vi "simple-LevyLab Analysis Framework (Template).vi"() -> ()   [LabVIEW 2019]
doc: "simple-LevyLab Analysis Framework (s-LLAF).\n\nDrag onto an empty block diagram to make your own."
uses:
  <vilib>/PRIrvin/XY Utilities/Typedefs/Interpolation Configuration--cluster.ctl
  <userlib>/LevyLab/LV-Data/LV-Data.ITX/Typedefs/Retrieve Data Type.ctl
  <vilib>/PRIrvin/Graph Utilities/graph_utilities.lvclass
  <userlib>/LevyLab/LV-Data/LV-Data/Typedefs/Dictionary--cluster.ctl
  <vilib>/PRIrvin/Graph Utilities/graph_utilities.lvclass/graph_utilities.ctl
  c6ffbd9c-2039-4b06-9ae2-0340eb0d4766.vi
  <vilib>/Analysis/baseanly.llb/Mean (DBL).vi
  4205ac38-1c06-43f0-93e0-ac3005b12872.vi
  <vilib>/Analysis/baseanly.llb/A x B.vi
  <vilib>/Analysis/baseanly.llb/A x Vector.vi
  <vilib>/PRIrvin/XY Utilities/subVIs/Square (single).vi
  <vilib>/PRIrvin/XY Utilities/subVIs/Sort (single).vi
  <vilib>/PRIrvin/XY Utilities/subVIs/Decimate (single).vi
  <vilib>/PRIrvin/XY Utilities/subVIs/Swap X and Y (single).vi
  <vilib>/PRIrvin/XY Utilities/subVIs/Reverse (single).vi
  <vilib>/PRIrvin/XY Utilities/subVIs/Subset (single).vi
  <vilib>/PRIrvin/XY Utilities/subVIs/Derivative (single).vi
  <vilib>/PRIrvin/XY Utilities/subVIs/Difference Quotient (single).vi
  <vilib>/PRIrvin/XY Utilities/subVIs/Interpolate (single).vi
  <vilib>/PRIrvin/XY Utilities/subVIs/FFT (single).vi
  <vilib>/PRIrvin/XY Utilities/subVIs/PS (single).vi
  <vilib>/PRIrvin/XY Utilities/subVIs/Moving Average (single).vi
  <vilib>/PRIrvin/XY Utilities/subVIs/Savitsky Golay Filter (single).vi
  <vilib>/PRIrvin/XY Utilities/subVIs/Zero Phase Lowpass Filter (single).vi
  <vilib>/PRIrvin/XY Utilities/subVIs/Symmetrize (single).vi
  <vilib>/Analysis/2dsp.llb/Decimate (single shot).vi
  <vilib>/Analysis/2dsp.llb/Decimate (single shot, DBL).vi
  <vilib>/Analysis/2dsp.llb/Derivative x(t).vi
  <vilib>/PRIrvin/XY Utilities/Private/X Array Index to Range.vi
  <vilib>/PRIrvin/XY Utilities/Private/X Units.vi
  <vilib>/PRIrvin/XY Utilities/Private/DQ subVI.vi
  <vilib>/PRIrvin/XY Utilities/subVIs/Divide float (single).vi
  <vilib>/PRIrvin/XY Utilities/subVIs/Add XY (single).vi
  <vilib>/PRIrvin/XY Utilities/subVIs/XY to Waveform (single).vi
  <vilib>/PRIrvin/XY Utilities/Private/Get X Array dx.vi
  <vilib>/Analysis/3filter.llb/Savitzky-Golay Filter.vi
  <vilib>/Analysis/3filter.llb/Savitzky-Golay Filter (DBL).vi
  <vilib>/PRIrvin/XY Utilities/Private/X Array Range to Index.vi
  <vilib>/PRIrvin/XY Utilities/subVIs/Get X and Y (single).vi
  <vilib>/PRIrvin/XY Utilities/subVIs/Resample (single).vi
  <vilib>/PRIrvin/Graph Utilities/XY Graph/Set XY Graph Value (array).vi
  <vilib>/PRIrvin/Graph Utilities/XY Graph/Get XY Graph Value.vi
  <vilib>/PRIrvin/Graph Utilities/Intensity Graph/Set Intensity Graph X Scale Array.vi
  <vilib>/PRIrvin/Graph Utilities/XY Graph/Get XY Graph X Label.vi
  <vilib>/PRIrvin/Graph Utilities/Intensity Graph/Set Intensity Graph X Label.vi
  <vilib>/PRIrvin/Graph Utilities/XY Graph/Get XY Graph Y Label.vi
  <vilib>/PRIrvin/Graph Utilities/Intensity Graph/Set Intensity Graph Z Label.vi
  <vilib>/PRIrvin/Graph Utilities/Intensity Graph/Set Intensity Graph Y Scale Array.vi
  <vilib>/PRIrvin/Graph Utilities/Intensity Graph/Set Intensity Graph Y Label.vi
  <vilib>/PRIrvin/Graph Utilities/Intensity Graph/Get Intensity Graph Cursor (Control).vi
  <vilib>/PRIrvin/Graph Utilities/Intensity Graph/Set Intensity Graph Cursor.vi
  <vilib>/PRIrvin/Graph Utilities/Intensity Graph/Get Intensity Graph X Scale.vi
  <vilib>/PRIrvin/Graph Utilities/Intensity Graph/Get Intensity Graph Value.vi
  <vilib>/PRIrvin/Graph Utilities/Intensity Graph/Get Intensity Graph Y Scale.vi
  <vilib>/PRIrvin/Graph Utilities/subVIs/Step Average.vi
  <vilib>/PRIrvin/Graph Utilities/subVIs/Normalized Gaussian.vi
  <vilib>/PRIrvin/Graph Utilities/Intensity Graph/Get Intensity Graph Y Label.vi
  <vilib>/PRIrvin/Graph Utilities/XY Graph/Set XY Graph X Label.vi
  <vilib>/PRIrvin/Graph Utilities/Intensity Graph/Get Intensity Graph Z Label.vi
  <vilib>/PRIrvin/Graph Utilities/XY Graph/Set XY Graph Y Label.vi
  <vilib>/PRIrvin/Graph Utilities/Intensity Graph/Get Intensity Graph X Label.vi
  <userlib>/_OpenG.lib/file/file.llb/Build Path - File Names Array__ogtk.vi
  <userlib>/_OpenG.lib/array/array.llb/Sort Array__ogtk.vi
  <userlib>/_OpenG.lib/array/array.llb/Sort 1D Array (DBL)__ogtk.vi
  <userlib>/_OpenG.lib/array/array.llb/Reorder Array2__ogtk.vi
  <userlib>/_OpenG.lib/array/array.llb/Reorder 1D Array2 (DBL)__ogtk.vi
  <userlib>/_MGI/1D Array/MGI Interpolate 1D Array Extended.vi
  <vilib>/Analysis/1siggen.llb/Ramp Pattern.vi
  <vilib>/Analysis/1siggen.llb/Ramp Pattern by Delta.vi
  <vilib>/gmath/interp.llb/Interpolate 1D.vi
  <vilib>/measure/maresamp.llb/Resample Waveforms (single shot).vi
  <vilib>/measure/maresamp.llb/Resample Pair of Arrays (single shot).vi
  <vilib>/measure/maspectr.llb/FFT Spectrum (Mag-Phase).vi
  <vilib>/measure/maspectr.llb/FFT Spectrum (Mag-Phase) for 1 Chan.vi
  <vilib>/measure/maspectr.llb/FFT Power Spectrum and PSD.vi
  <vilib>/measure/maspectr.llb/FFT Power Spectrum and PSD for 1 Chan.vi
  <vilib>/measure/maresamp.llb/Resample N Pairs of Arrays (single shot).vi
  <vilib>/ptbypt/Probability & Statistics.llb/Mean PtByPt.vi
  <vilib>/Analysis/3filter.llb/FIR Windowed Coefficients.vi
  <vilib>/Analysis/3filter.llb/Zero Phase Filter.vi
  <vilib>/Analysis/3filter.llb/Zero Phase Filter (DBL).vi
  <vilib>/PRIrvin/XY Utilities/xy_utilities.lvlib
  <userlib>/LevyLab/LV-Data/LV-Data/LV-Data.lvclass
  <userlib>/LevyLab/LV-Data/LV-Data.ITX/LV-Data.ITX.lvclass
  <vilib>/Analysis/NI_AALBase.lvlib
  <userlib>/LevyLab/LV-Data/LV-Data/API/XY-Data to Dictionary (single).vi
  <vilib>/PRIrvin/XY Utilities/subVIs/Subtract float (single).vi
  <vilib>/PRIrvin/XY Utilities/subVIs/Add float (single).vi
  <vilib>/PRIrvin/XY Utilities/subVIs/Waveform to XY (single).vi
  <vilib>/PRIrvin/XY Utilities/subVIs/Multiply float (single).vi
  <vilib>/PRIrvin/XY Utilities/subVIs/Restrict X Range (single).vi
  <vilib>/PRIrvin/XY Utilities/subVIs/Interpolate Y (single).vi
  <vilib>/PRIrvin/XY Utilities/subVIs/Log (single).vi
  <vilib>/PRIrvin/XY Utilities/subVIs/Linear Fit (multiple).vi
  <vilib>/PRIrvin/XY Utilities/subVIs/Append (multiple).vi
  <vilib>/PRIrvin/XY Utilities/subVIs/Shift Zero (single).vi
  <vilib>/PRIrvin/XY Utilities/subVIs/Peak Detector (single).vi
  <vilib>/PRIrvin/XY Utilities/subVIs/Remove Outliers (single).vi
  a4d1e059-db4b-46df-9b26-41dcdcc29953.vi
  8d1aee34-a274-4619-8160-c9a8fc862039.vi
  eec88c9d-a91b-41fb-93d9-32a34acbf560.vi
  a819f7a0-c833-4e57-b12c-b555cdea62a2.vi
  2a0ce4de-3a5e-4348-8ae1-e372722f1305.vi
  8311829f-ef70-43ef-acfd-10b322ed8a94.vi
  <vilib>/PRIrvin/XY Utilities/subVIs/Add float (multiple).vi
  <vilib>/PRIrvin/XY Utilities/subVIs/Subtract float (multiple).vi
  <vilib>/PRIrvin/XY Utilities/subVIs/Multiply float (multiple).vi
  <vilib>/PRIrvin/XY Utilities/subVIs/Square (multiple).vi
  <vilib>/PRIrvin/XY Utilities/subVIs/Divide float (multiple).vi
  <vilib>/PRIrvin/XY Utilities/subVIs/Sort (multiple).vi
  <vilib>/PRIrvin/XY Utilities/subVIs/Decimate (multiple).vi
  <vilib>/PRIrvin/XY Utilities/subVIs/Swap X and Y (multiple).vi
  <vilib>/PRIrvin/XY Utilities/subVIs/Reverse (multiple).vi
  <vilib>/PRIrvin/XY Utilities/subVIs/Subset (multiple).vi
  <vilib>/PRIrvin/XY Utilities/subVIs/Derivative (multiple).vi
  <vilib>/PRIrvin/XY Utilities/subVIs/Difference Quotient (multiple).vi
  <vilib>/PRIrvin/XY Utilities/subVIs/Interpolate (multiple).vi
  <vilib>/PRIrvin/XY Utilities/subVIs/FFT (multiple).vi
  <vilib>/PRIrvin/XY Utilities/subVIs/PS (multiple).vi
  <vilib>/PRIrvin/XY Utilities/subVIs/Resample (multiple).vi
  <vilib>/PRIrvin/XY Utilities/subVIs/Moving Average (multiple).vi
  <vilib>/PRIrvin/XY Utilities/subVIs/Savitsky Golay Filter (multiple).vi
  <vilib>/PRIrvin/XY Utilities/subVIs/Zero Phase Lowpass Filter (multiple).vi
  <vilib>/PRIrvin/XY Utilities/subVIs/Symmetrize (multiple).vi
panel:
  out "time (ms)":dbl
  in  "Tab Control":enum32{"Load Data", "Help"}(tab)
  in  "regex after":string
  in  "param in notes":bool
  in  "list recursive":bool
  in  "Path":path
  out "Notes":string
  in  "Data Type":T1=enum."DAT"
  in  "SAVE":bool
  in  "PROCESS":bool
  in  "CLEAR":bool
  in  "LOAD":bool
  in  "Z":u16(ring) items=["Delay", "Temperature", "Time", "Ch1_x", "Ch1_y", "Ch1_PS_x", "Ch1_PS_y", "Ch2_x", "Ch2_y", "Ch2_PS_x", "Ch2_PS_y", "Ch3_x", "Ch3_y", "Ch3_PS_x", "Ch3_PS_y", "Ch4_x", "Ch4_y", "Ch4_PS_x", "Ch4_PS_y", "Ch5_x", "Ch5_y", "Ch5_PS_x", "Ch5_PS_y", "Ch6_x", "Ch6_y", "Ch6_PS_x", "Ch6_PS_y", "Ch7_x", "Ch7_y", "Ch7_PS_x", "Ch7_PS_y", "Ch8_x", "Ch8_y", "Ch8_PS_x", "Ch8_PS_y"]
  in  "Y":u16(ring) items=["Delay", "Temperature", "Time", "Ch1_x", "Ch1_y", "Ch1_PS_x", "Ch1_PS_y", "Ch2_x", "Ch2_y", "Ch2_PS_x", "Ch2_PS_y", "Ch3_x", "Ch3_y", "Ch3_PS_x", "Ch3_PS_y", "Ch4_x", "Ch4_y", "Ch4_PS_x", "Ch4_PS_y", "Ch5_x", "Ch5_y", "Ch5_PS_x", "Ch5_PS_y", "Ch6_x", "Ch6_y", "Ch6_PS_x", "Ch6_PS_y", "Ch7_x", "Ch7_y", "Ch7_PS_x", "Ch7_PS_y", "Ch8_x", "Ch8_y", "Ch8_PS_x", "Ch8_PS_y"]
  in  "A":u16(ring) items=["Delay", "Temperature", "Time", "Ch1_x", "Ch1_y", "Ch1_PS_x", "Ch1_PS_y", "Ch2_x", "Ch2_y", "Ch2_PS_x", "Ch2_PS_y", "Ch3_x", "Ch3_y", "Ch3_PS_x", "Ch3_PS_y", "Ch4_x", "Ch4_y", "Ch4_PS_x", "Ch4_PS_y", "Ch5_x", "Ch5_y", "Ch5_PS_x", "Ch5_PS_y", "Ch6_x", "Ch6_y", "Ch6_PS_x", "Ch6_PS_y", "Ch7_x", "Ch7_y", "Ch7_PS_x", "Ch7_PS_y", "Ch8_x", "Ch8_y", "Ch8_PS_x", "Ch8_PS_y"]
  in  "C":u16(ring) items=["Delay", "Temperature", "Time", "Ch1_x", "Ch1_y", "Ch1_PS_x", "Ch1_PS_y", "Ch2_x", "Ch2_y", "Ch2_PS_x", "Ch2_PS_y", "Ch3_x", "Ch3_y", "Ch3_PS_x", "Ch3_PS_y", "Ch4_x", "Ch4_y", "Ch4_PS_x", "Ch4_PS_y", "Ch5_x", "Ch5_y", "Ch5_PS_x", "Ch5_PS_y", "Ch6_x", "Ch6_y", "Ch6_PS_x", "Ch6_PS_y", "Ch7_x", "Ch7_y", "Ch7_PS_x", "Ch7_PS_y", "Ch8_x", "Ch8_y", "Ch8_PS_x", "Ch8_PS_y"]
  in  "B":u16(ring) items=["Delay", "Temperature", "Time", "Ch1_x", "Ch1_y", "Ch1_PS_x", "Ch1_PS_y", "Ch2_x", "Ch2_y", "Ch2_PS_x", "Ch2_PS_y", "Ch3_x", "Ch3_y", "Ch3_PS_x", "Ch3_PS_y", "Ch4_x", "Ch4_y", "Ch4_PS_x", "Ch4_PS_y", "Ch5_x", "Ch5_y", "Ch5_PS_x", "Ch5_PS_y", "Ch6_x", "Ch6_y", "Ch6_PS_x", "Ch6_PS_y", "Ch7_x", "Ch7_y", "Ch7_PS_x", "Ch7_PS_y", "Ch8_x", "Ch8_y", "Ch8_PS_x", "Ch8_PS_y"]
  in  "X":u16(ring) items=["Delay", "Temperature", "Time", "Ch1_x", "Ch1_y", "Ch1_PS_x", "Ch1_PS_y", "Ch2_x", "Ch2_y", "Ch2_PS_x", "Ch2_PS_y", "Ch3_x", "Ch3_y", "Ch3_PS_x", "Ch3_PS_y", "Ch4_x", "Ch4_y", "Ch4_PS_x", "Ch4_PS_y", "Ch5_x", "Ch5_y", "Ch5_PS_x", "Ch5_PS_y", "Ch6_x", "Ch6_y", "Ch6_PS_x", "Ch6_PS_y", "Ch7_x", "Ch7_y", "Ch7_PS_x", "Ch7_PS_y", "Ch8_x", "Ch8_y", "Ch8_PS_x", "Ch8_PS_y"]
  in  "regex before":string
  in  "Action Tab Control":enum32{"Page 1", "Page 2"}(tab)
  out "Processed States":string="XY: Load\nGraph: Initialize Graphs\nUI: Display Data"
  in  "Available States":i32(listbox)=-1 caption="States to Process"
  in  "Process Queue":string
  out "Current State":string
  in  "Type":enum16{"y/x vs x", "x/y vs y"}(ring)
  in  "Window":dbl=2.0
  in  "Units":enum16{"Points", "Data"}(ring)
  in  "Configure":T2={"X Low"=0.05, "X High"=0.5, "X Step"=0.01, "Fake Point"=0.05} {"Fake Point" format="%#_6p"; "X Step" format="%#_6p"; "X High" format="%#_6p"; "X Low" format="%#_6p"}
  in  "y":dbl format="%#_6p"
  in  "x":dbl format="%#_6p"
  in  "Type":enum16{"dy/dx vs x", "dx/dy vs y"}(ring)
  in  "Subset Slider":cluster{dbl, dbl}(slide)={0.75, 0.25} caption="Horizontal Slider" scale=0.0..1.0
  in  "Method":enum16{"Slider (%)", "X[] min and max"}(ring)
  in  "SG side points":dbl
  in  "Moving Window":dbl=5000.0 format="%#_13g"
  in  "Zero Phase cutoff":dbl
  in  "decimating factor":i32=1
  in  "averaging":bool
  in  "Graphs Tab Control":enum32{"Data", "Intensity/Linecuts"}(tab)
  out "XY Graph: Antisymmetric":cluster{"X-array":dbl[], dbl[]}[](graph)
  out "XY Graph: Processed":cluster{"Intensity Data":dbl[], "Array":dbl[]}[](graph)
  out "XY Graph: Unprocessed":cluster{"Intensity Data":dbl[], "Array":dbl[]}[](graph)
  out "XY Graph: Symmetric":cluster{"X-array":dbl[], dbl[]}[](graph)
  out "Data Intensity":dbl[][](graph)
  out "Diff Intensity":dbl[][](graph)
  out "Diff Vertical":cluster{"Array":dbl[], "A x Vector":dbl[]}[](graph)
  out "Diff Horizontal":cluster{"Array":dbl[], "A x Vector":dbl[]}[](graph)
  in  "width (vertical)":dbl=0.2 caption="width"
  in  "width (horizontal)":dbl=0.2 caption="width"
  in  "width (vertical) 2":dbl=0.2 caption="width"
  in  "width (horizontal) 2":dbl=0.2 caption="width"
  out "Data Vertical":cluster{"Array":dbl[], "A x Vector":dbl[]}[](graph)
  out "Data Horizontal":cluster{"Intensity Data":dbl[], "Array":dbl[]}[](graph)
  in  "Color Map":T3(ring)=enum."Viridis"
  in  "Color Map 2":T3(ring)=enum."Viridis"
  # "Load Data"
  # "Actions"
  # "Load Data:\n- \"Path\" can be a file or a folder; \"TDMS Groups\" will read this many groups from a single file\n- A,B,C refer to the 1st, 2nd, 3rd datasets to read from the file. They are combined in the state \"Data: Select Channels\" to calculate, for example Rxx or Rxy\n- X, Y, Z are independent vaiables (eg, X = Vsg, Y = Magnet)\nState Scripting:\n- \"Process Queue\" is a list of states that will execute when you press the \"PROCESS\" button. (File: Load and Graph: Update Graph are added automatically to the beginning and end of the queue.)\nTo add states you can either:\n- Type directly into the Process Queue box.\nor:\n- Select a state in the \"Available States\" box that you want to add to the queue. ctl-v in the \"Process Queue\" control to add to the queue."
  # "State Scripting"
  # "Process Arguments"
  # "Arithmetic"
  # "Interpolate"
  # "Subset"
  # "Filters"
  # "Derivative"
  # "Difference Quotient"
  # "XY Graphs"
  # "Symmeterized Graphs"
  # "Data processing (1)"
  # "Data Processing (2)"
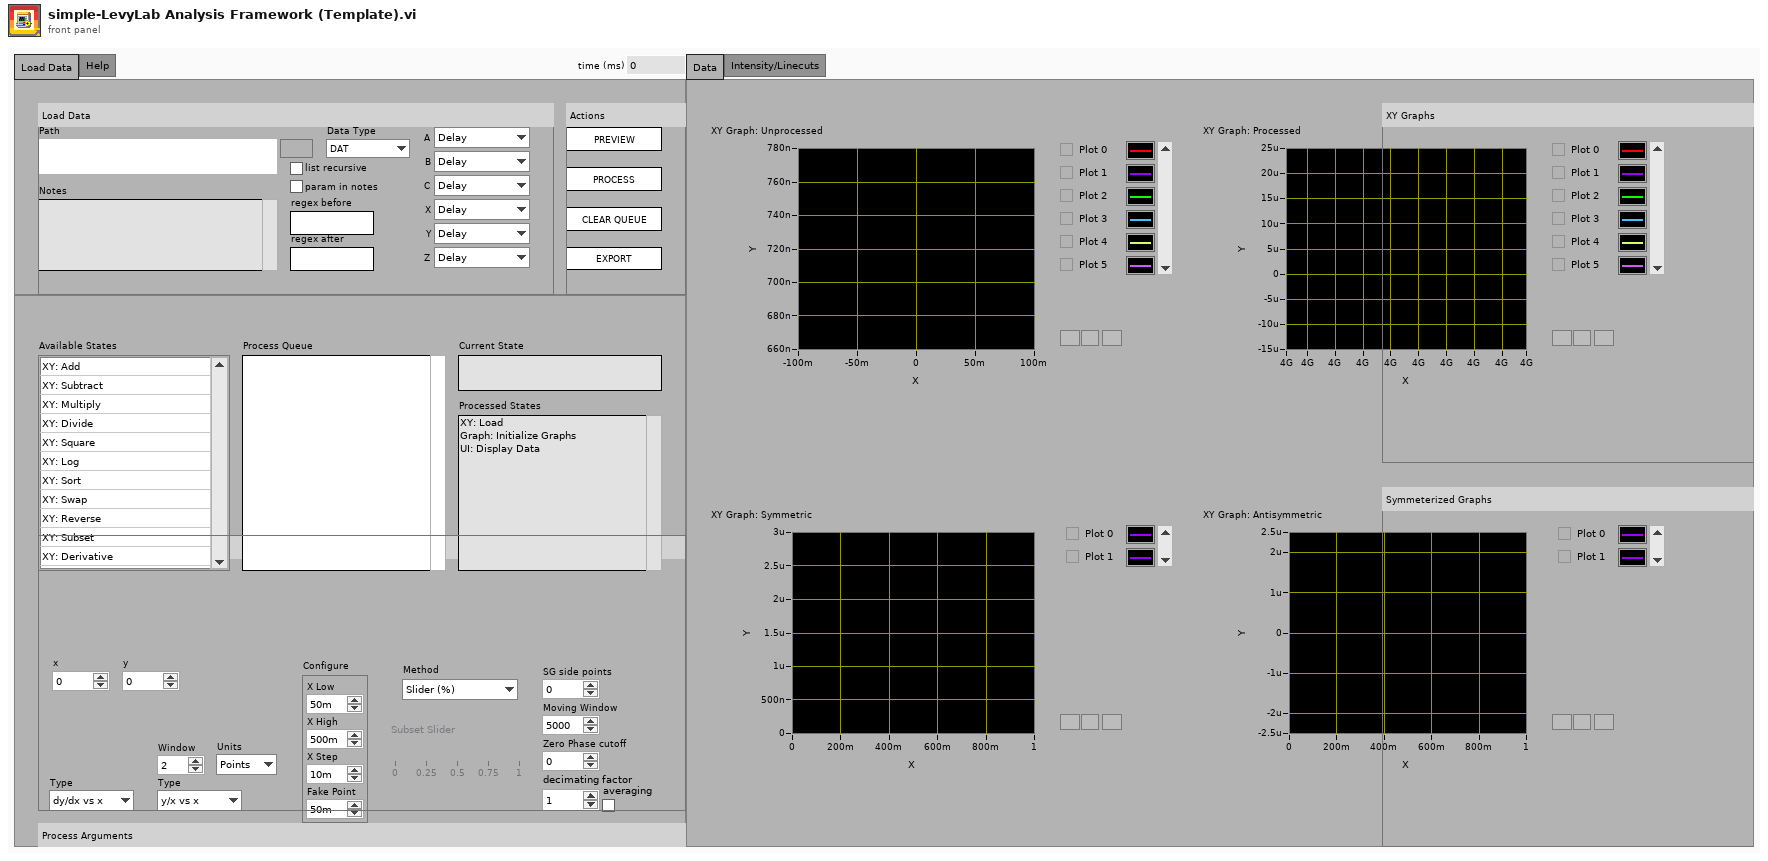
[diagram p1: front panel]
types:
  T1 = typedef "LV-Data.ITX.lvclass/Retrieve Data Type.ctl" = enum16{"ITX", "ITX w/ 2D", "DAT", "TDMS"}
  T2 = typedef "xy_utilities.lvlib/Interpolation Configuration--cluster.ctl" = cluster{"X Low":dbl, "X High":dbl, "X Step":dbl, "Fake Point":dbl}
  T3 = enum16{"Inferno", "Kindlmann", "Plasma", "Viridis", "LevyLab2010", "ColorCET...", "Custom..."}
  T4 = enum32{"Invalid", "Standard", "Closed", "Hidden", "Minimized", "Maximized"}
  T5 = enum32{"invalid app kind", "Development System", "Run Time System", "Student Edition", "Embedded LabVIEW", "Evaluation", "Custom"}
  T6 = typedef "LV-Data.lvclass/Dictionary--cluster.ctl" = cluster{"key":string, "value":variant}
  T7 = cluster{"Core":cluster{"Current VI Reference":refnum<vi>, "Close Panel on Exit?":bool}, "Path":path, "Paths":path[], "Graph":cluster{"Data: Unprocessed":refnum<class "graph_utilities.lvclass">, "Data: Processed":refnum<class "graph_utilities.lvclass">, "Data: Intensity/Vertical":refnum<class "graph_utilities.lvclass">, "Data: Intensity/Horizontal":refnum<class "graph_utilities.lvclass">, "Differential: Intensity/Vertical":refnum<class "graph_utilities.lvclass">, "Differential: Intensity/Horizontal":refnum<class "graph_utilities.lvclass">}, "Rings":cluster{"X":refnum<vi>, "Y":refnum<vi>, "Z":refnum<vi>, "A":refnum<vi>, "B":refnum<vi>, "C":refnum<vi>}, "Dictionaries":cluster{"Data (Dictionary)":T6[]}[], "Keys":cluster{"X":string, "Y":string, "Z":string, "A":string, "B":string, "C":string}, "XY Data (unprocessed)":cluster{"X-array":dbl[], "Y-array":dbl[]}[], "XY Data (processed 1)":cluster{"X-array":dbl[], "Y-array":dbl[]}[], "XY Data (processed 2)":cluster{"X-array":dbl[], "Y-array":dbl[]}[], "Parameter":dbl[]}
  T8 = cluster{"Shift":bool, "Ctrl":bool, "Alt":bool, "Cmd":bool, "Opt":bool}
  T9 = cluster{"X":string, "Y":string, "Z":string, "A":string, "B":string, "C":string}
  T10 = cluster{"X":refnum<vi>, "Y":refnum<vi>, "Z":refnum<vi>, "A":refnum<vi>, "B":refnum<vi>, "C":refnum<vi>}
  T11 = cluster{"Data: Unprocessed":refnum<class "graph_utilities.lvclass">, "Data: Processed":refnum<class "graph_utilities.lvclass">, "Data: Intensity/Vertical":refnum<class "graph_utilities.lvclass">, "Data: Intensity/Horizontal":refnum<class "graph_utilities.lvclass">, "Differential: Intensity/Vertical":refnum<class "graph_utilities.lvclass">, "Differential: Intensity/Horizontal":refnum<class "graph_utilities.lvclass">}
  T12 = cluster{"Current VI Reference":refnum<vi>, "Close Panel on Exit?":bool}
  T13 = typedef "LV-Data.lvclass/Map Variant--map.ctl" = map{string, variant}
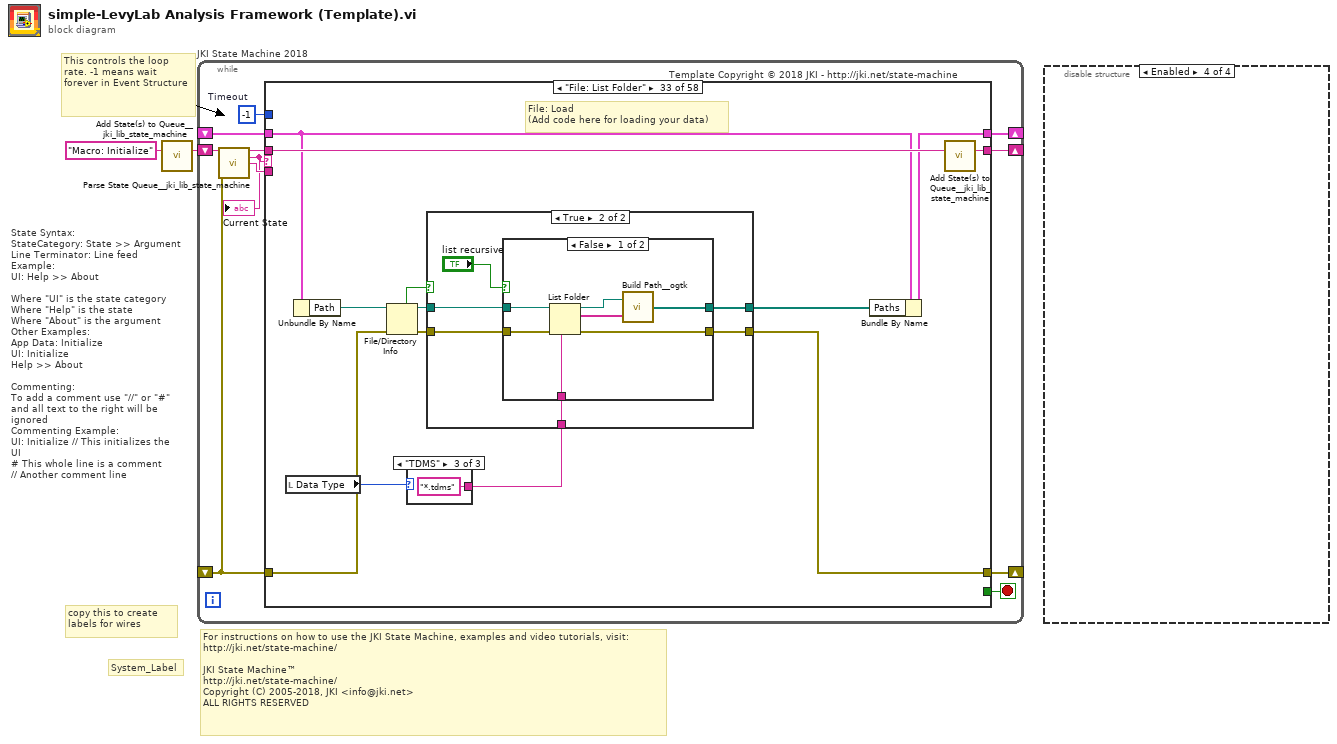
[diagram p0: block diagram]
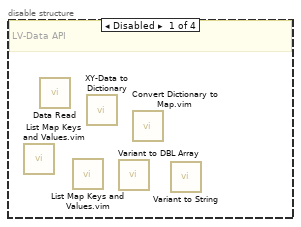
[diagram p2: hidden frame]
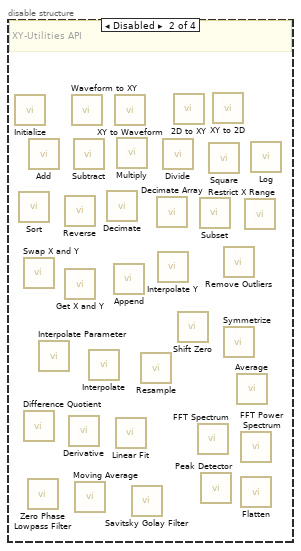
[diagram p3: hidden frame]
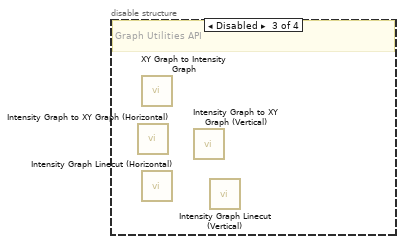
[diagram p4: hidden frame]
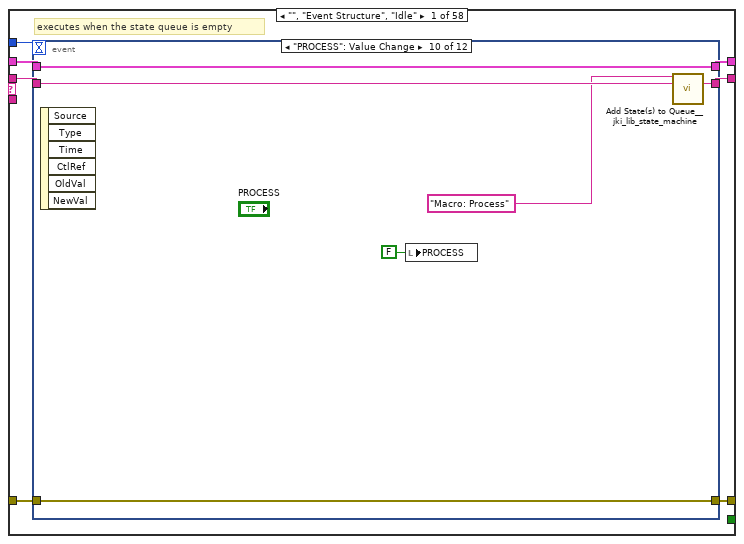
[diagram p5: hidden frame]
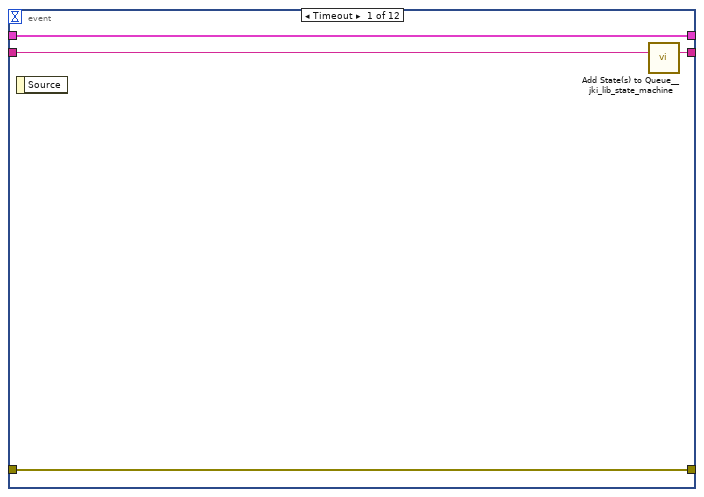
[diagram p6: hidden frame]
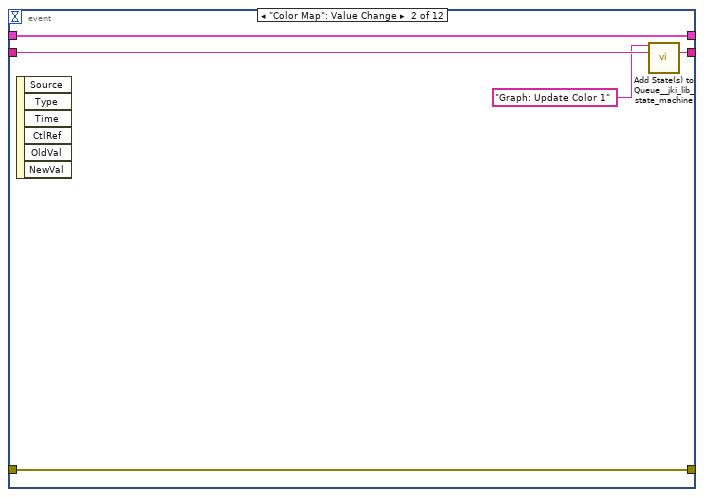
[diagram p7: hidden frame]
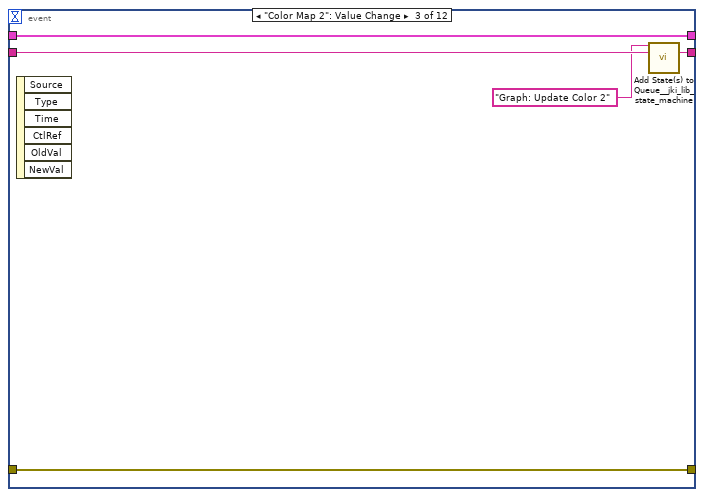
[diagram p8: hidden frame]
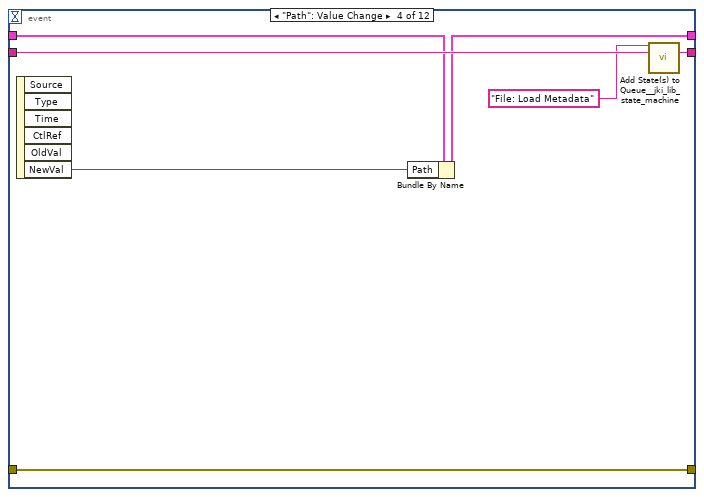
[diagram p9: hidden frame]
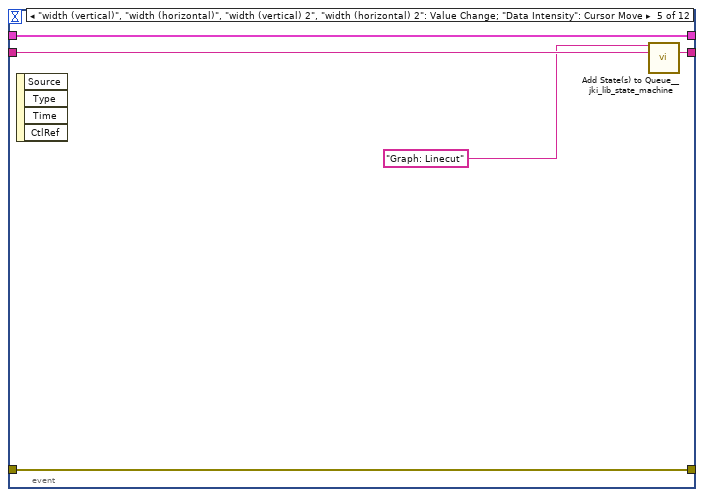
[diagram p10: hidden frame]
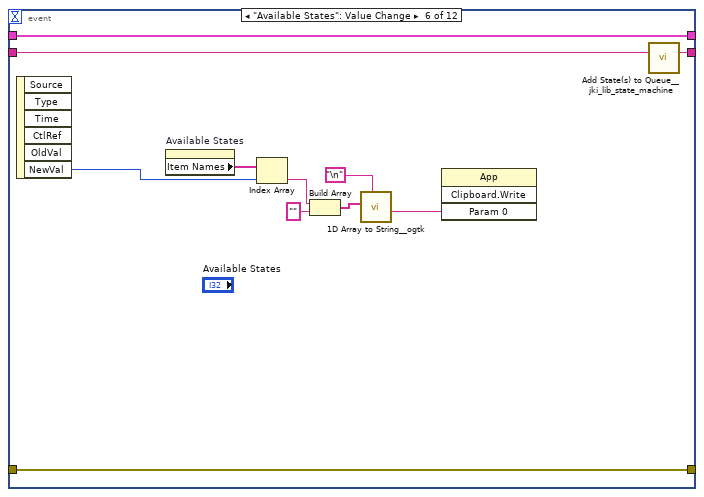
[diagram p11: hidden frame]
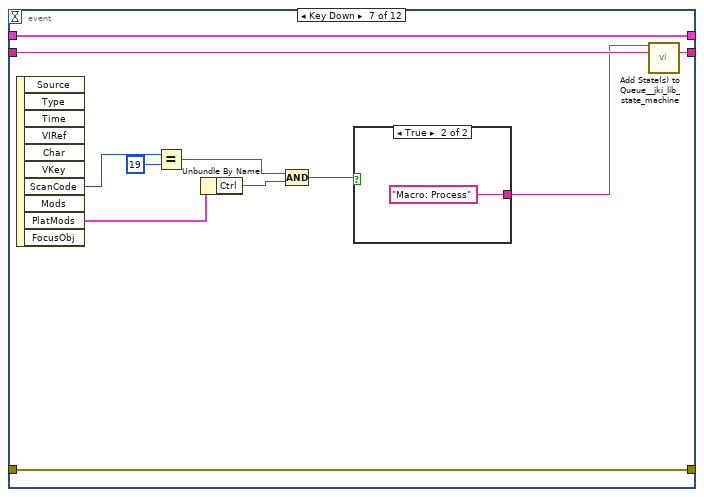
[diagram p12: hidden frame]
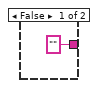
[diagram p13: hidden frame]
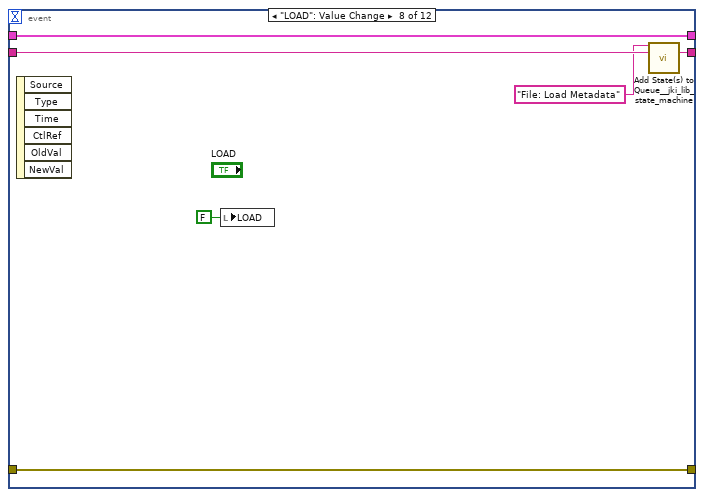
[diagram p14: hidden frame]
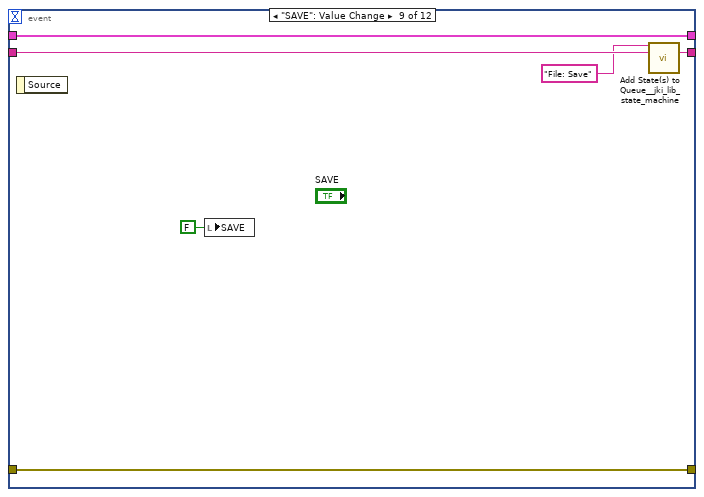
[diagram p15: hidden frame]
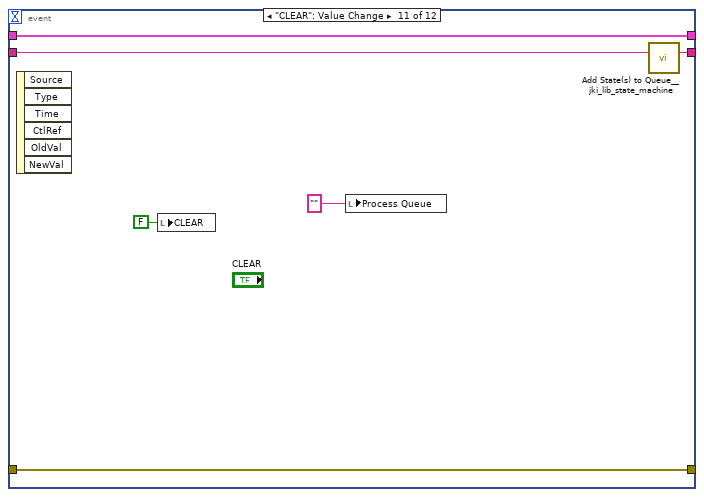
[diagram p16: hidden frame]
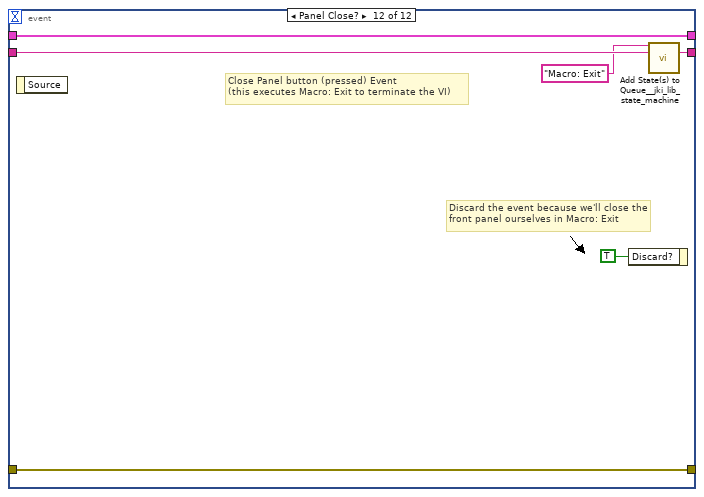
[diagram p17: hidden frame]
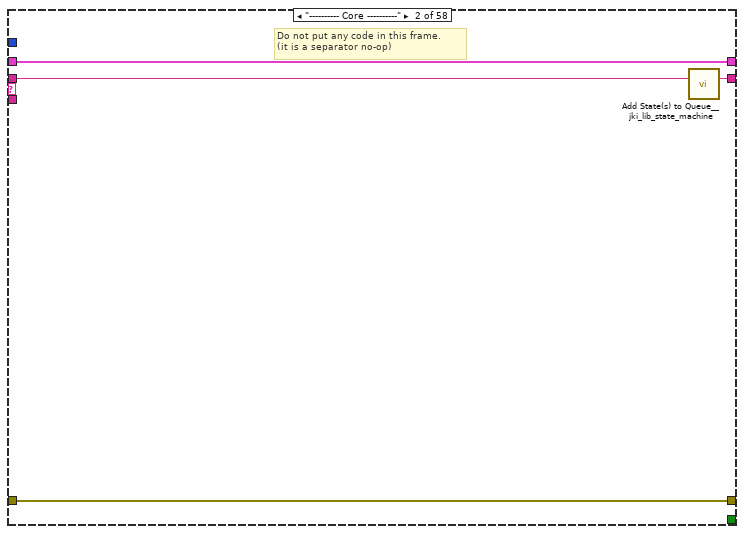
[diagram p18: hidden frame]
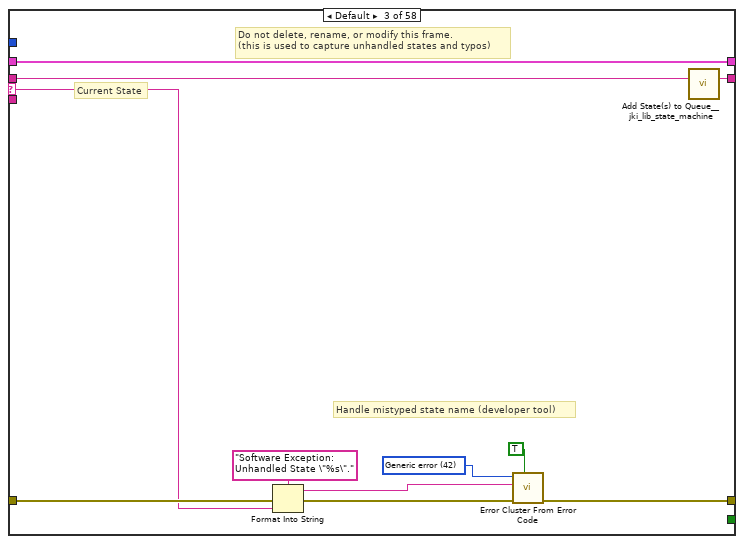
[diagram p19: hidden frame]
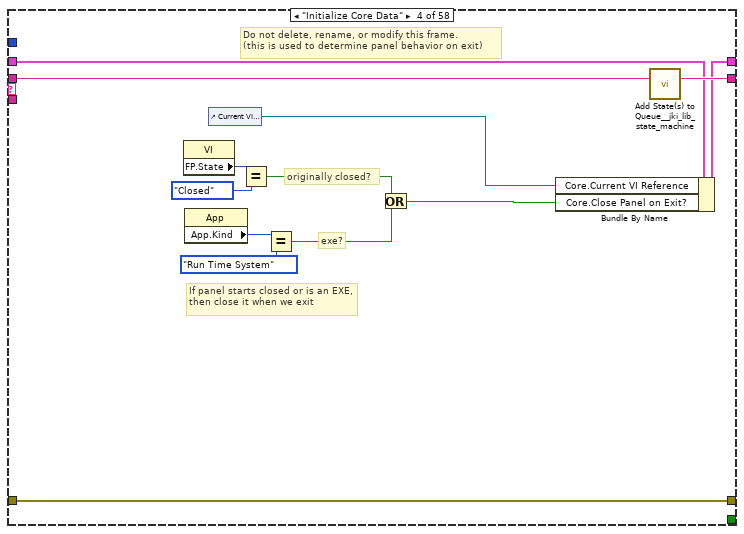
[diagram p20: hidden frame]
diagram:
  # "For instructions on how to use the JKI State Machine, examples and video tutorials, visit:\nhttp://jki.net/state-machine/\n\nJKI State Machine™\nhttp://jki.net/state-machine/\nCopyright (C) 2005-2018, JKI <info@jki.net>\nALL RIGHTS RESERVED"
  # "State Syntax:\nStateCategory: State >> Argument\nLine Terminator: Line feed\nExample:\nUI: Help >> About\n\nWhere \"UI\" is the state category\nWhere \"Help\" is the state\nWhere \"About\" is the argument\nOther Examples:\nApp Data: Initialize\nUI: Initialize\nHelp >> About\n\nCommenting:\nTo add a comment use \"//\" or \"#\" and all text to the right will be ignored\nCommenting Example:\nUI: Initialize // This initializes the UI\n# This whole line is a comment\n// Another comment line"
  # "copy this to create labels for wires"
  # "This controls the loop rate. -1 means wait forever in Event Structure"
  # "System_Label"
  n1 = call <vilib>:"Add State(s) to Queue__jki_lib_state_machine.vi"("State(s) in (\"\")"="Macro: Initialize") -> ("States Out"=w2:string)  [unwired: 14 in]
  n2 = while "JKI State Machine 2018" {
    shift-right: [w7] -> _
    shift-left: _ -> [w6]
    shift-right: [w10] -> _
    shift-left: _ -> [w4]
    shift-right: [w9] -> _
    shift-left: w2 -> [w11]
    stop <- w8 stop-if-true
    w5 = -1  # Timeout
    # "Template Copyright © 2018 JKI - http://jki.net/state-machine"
    n3 = call <vilib>:"Parse State Queue__jki_lib_state_machine.vi"("State Queue"=w11, "Error In (no error)"=w4) -> ("Remaining States"=w13:string, "Current State"=w3:string, "Arguments"=w12:string)  [unwired: 11 in]
    "Current State" <- w3
    n4 = case shown="\"File: List Folder\"" w3 {
      selector: w3 -> [_ _ w105 _ _ _ _ _ _ _ _ _ _ _ _ _ _ _ _ _ _ _ _ _ _ _ _ _ _ _ _ _ _ _ _ _ _ _ _ _ _ _ _ _ _ _ _ _ _ _ _ _ _ _ _ _ _ _]
      tunnel: w13 -> [w20 w104 w109 w128 w134 w139 w143 w158 w173 w191 w226 w230 w242 w248 w259 w328 w333 w343 w353 w357 w361 w378 w402 w413 w423 w450 w485 w501 w509 w517 w521 w538 w579 w614 w653 w661 w671 w681 w691 w699 w706 w720 w728 w738 w746 w754 w765 w778 w789 w798 w806 w814 w822 w830 w839 w848 w857 w867]
      tunnel: w12 -> [_ _ _ _ _ _ _ _ _ _ _ _ _ w243 w253 _ _ _ _ _ _ _ _ _ _ _ _ _ _ _ _ _ _ _ _ _ _ _ _ _ _ _ _ _ _ _ w755 _ _ _ _ _ _ _ _ _ _ _]
      tunnel: w6 -> [w18 w101 w107 w121 w131 w137 w140 _ w166 w187 w221 w227 w240 w246 w255 w325 w330 w340 w350 w354 w358 w376 w400 w409 w420 w448 w482 w499 w507 w515 w518 w536 w576 w611 w650 w658 w668 w678 w688 w696 w704 w717 w725 w735 w743 w751 w762 w775 w786 w795 w803 w811 w819 w827 w836 w845 w854 w864]
      tunnel: [w17 w102 w111 w125 errorcluster {"status"=FALSE, "code"=0, "source"=""} ("error out") w136 w141 w155 w160 w186 w222 w228 w233 w244 w256 w326 w331 w341 w351 w355 w359 w374 w385 w411 w418 w440 w483 w490 w503 w512 w519 w530 w568 w605 w648 w654 w664 w674 w684 w692 w702 w713 w721 w731 w739 w747 w758 w772 w783 w791 w799 w808 w815 w823 w832 w841 w850 w860] -> w10
      tunnel: w4 -> [w16 w102 w110 w125 w130 w136 w141 w155 w168 w183 w223 w228 w234 w245 w257 w326 w331 w341 w351 w355 w359 w365 w379 w411 w419 w443 w483 w492 w502 w511 w519 w526 w574 w606 w647 w655 w665 w675 w685 w693 w702 w714 w722 w732 w740 w748 w759 w773 w784 w792 w800 w809 w816 w824 w833 w842 w851 w861]
      tunnel: [w19 w103 w108 w127 w133 w138 w142 w157 w172 w190 w225 w229 w241 w247 w258 w327 w332 w342 w352 w356 w360 w377 w401 w412 w422 w449 w484 w500 w508 w516 w520 w537 w578 w613 w652 w660 w670 w680 w690 w698 w705 w719 w727 w737 w745 w753 w764 w777 w788 w797 w805 w813 w821 w829 w838 w847 w856 w866] -> w9
      tunnel: [_ _ _ _ _ TRUE _ _ _ _ _ _ _ _ _ _ _ _ _ _ _ _ _ _ _ _ _ _ _ _ _ _ _ _ _ _ _ _ _ _ _ _ _ _ _ _ _ _ _ _ _ _ _ _ _ _ _ _] -> w8
      tunnel: [w15 w101 w107 w126 w131 w137 w140 w156 w167 w188 w221 w227 w240 w246 w255 w325 w330 w340 w350 w354 w358 w375 w399 w410 w420 w448 w482 w499 w507 w515 w518 w536 w577 w612 w650 w657 w667 w677 w687 w695 w703 w716 w724 w734 w742 w750 w761 w774 w785 w794 w802 w810 w818 w826 w835 w844 w853 w863] -> w7
      tunnel: w5 -> [w14 _ _ _ _ _ _ _ _ _ _ _ _ _ _ _ _ _ _ _ _ _ _ _ _ _ _ _ _ _ _ _ _ _ _ _ _ _ _ _ _ _ _ _ _ _ _ _ _ _ _ _ _ _ _ _ _ _]
      frame "", "Event Structure", "Idle" {
        # "executes when the state queue is empty"
        n5 = event shown="[9] \"PROCESS\": Value Change" {
          selector: _ -> [_ _ _ _ _ _ _ _ _ _ _ _]
          dyn-events: _ -> [_ _ _ _ _ _ _ _ _ _ _ _]
          timeout: w14 -> [_ _ _ _ _ _ _ _ _ _ _ _]
          tunnel: w20 -> [w24 w29 w34 w41 w46 w57 w68 w76 w82 w88 w94 w100]
          tunnel: [w23 w28 w33 w40 w45 w56 w67 w75 w81 w87 w93 w99] -> w19
          tunnel: w18 -> [w21 w26 w31 w37 w43 w54 w65 w73 w79 w85 w91 w97]
          tunnel: [w22 w27 w32 w39 w44 w55 w66 w74 w80 w86 w92 w98] -> w17
          tunnel: w16 -> [w22 w27 w32 w39 w44 w55 w66 w74 w80 w86 w92 w98]
          tunnel: [w21 w26 w31 w38 w43 w54 w65 w73 w79 w85 w91 w97] -> w15
          event Timeout {
            n6 = event-data() -> ()  [unwired: 1 in, 1 out]
            n7 = call <vilib>:"Add State(s) to Queue__jki_lib_state_machine.vi"("State(s) in (\"\")"=w24) -> ("States Out"=w23:string)  [unwired: 14 in]
          }
          event "Color Map": Value Change {
            n8 = event-data() -> ()  [unwired: 1 in, 6 out]
            n9 = call <vilib>:"Add State(s) to Queue__jki_lib_state_machine.vi"("State(s) in Front (\"\")"="Graph: Update Color 1" ("State(s) in Front (\"\")"), "State(s) in (\"\")"=w29) -> ("States Out"=w28:string)  [unwired: 13 in]
          }
          event "Color Map 2": Value Change {
            n10 = event-data() -> ()  [unwired: 1 in, 6 out]
            n11 = call <vilib>:"Add State(s) to Queue__jki_lib_state_machine.vi"("State(s) in Front (\"\")"="Graph: Update Color 2" ("State(s) in Front (\"\")"), "State(s) in (\"\")"=w34) -> ("States Out"=w33:string)  [unwired: 13 in]
          }
          event "Path": Value Change {
            n12 = event-data() -> ("NewVal"=w36:path)  [unwired: 1 in, 5 out]
            n13 = Bundle By Name(cluster=w37, "Path"=w36) -> (w38:T7)
            n14 = call <vilib>:"Add State(s) to Queue__jki_lib_state_machine.vi"("State(s) in Front (\"\")"="File: Load Metadata" ("State(s) in Front (\"\")"), "State(s) in (\"\")"=w41) -> ("States Out"=w40:string)  [unwired: 13 in]
          }
          event "width (vertical)", "width (horizontal)", "width (vertical) 2", "width (horizontal) 2": Value Change; "Data Intensity": Cursor Move {
            n15 = event-data() -> ()  [unwired: 1 in, 4 out]
            n16 = call <vilib>:"Add State(s) to Queue__jki_lib_state_machine.vi"("State(s) in Front (\"\")"="Graph: Linecut" ("State(s) in Front (\"\")"), "State(s) in (\"\")"=w46) -> ("States Out"=w45:string)  [unwired: 13 in]
          }
          event "Available States": Value Change {
            n17 = event-data() -> ("NewVal"=w48:i32)  [unwired: 1 in, 5 out]
            n18 = property on="Available States" class="LstBox (strict)"() -> ("Item Names"=w49:string[])  [unwired: 2 in, 2 out]
            n19 = Index Array(array=w49, index=w48) -> (element=w53:string)
            n20 = Build Array(w53, "" ("element")) -> (w50:string[])
            n21 = call <userlib>:"1D Array to String__ogtk.vi"("delimiter (Tab)"="\n", "Array of Strings"=w50) -> ("delimited string"=w51:string)  [unwired: 9 in]
            n22 = invoke class="App" method="Clipboard.Write"("Param 0"=w51) -> ()  [unwired: 3 in, 4 out]
            n23 = call <vilib>:"Add State(s) to Queue__jki_lib_state_machine.vi"("State(s) in (\"\")"=w57) -> ("States Out"=w56:string)  [unwired: 14 in]
          }
          event Key Down {
            n24 = event-data() -> ("ScanCode"=w58:i16, "PlatMods"=w59:T8)  [unwired: 1 in, 8 out]
            n25 = Equal?(x=w58, y=i16 19) -> (x = y?=w61:bool)
            n26 = Unbundle By Name(w59) -> ("Ctrl"=w62:bool)
            n27 = Compound Arithmetic op=AND(w61, w62) -> (w60:bool)
            n28 = case shown="True" w60 {
              tunnel: ["" ("State(s) in Front (\"\")") "Macro: Process" ("State(s) in Front (\"\")")] -> w63
              frame False {
              }
              frame True {
              }
            }
            n29 = call <vilib>:"Add State(s) to Queue__jki_lib_state_machine.vi"("State(s) in Front (\"\")"=w63, "State(s) in (\"\")"=w68) -> ("States Out"=w67:string)  [unwired: 13 in]
          }
          event "LOAD": Value Change {
            n30 = event-data() -> ()  [unwired: 1 in, 6 out]
            n31 = local write "LOAD"(FALSE ("LOAD")) -> ()
            n32 = call <vilib>:"Add State(s) to Queue__jki_lib_state_machine.vi"("State(s) in Front (\"\")"="File: Load Metadata" ("State(s) in Front (\"\")"), "State(s) in (\"\")"=w76) -> ("States Out"=w75:string)  [unwired: 13 in]
          }
          event "SAVE": Value Change {
            n33 = event-data() -> ()  [unwired: 1 in, 1 out]
            n34 = local write "SAVE"(FALSE ("SAVE")) -> ()
            n35 = call <vilib>:"Add State(s) to Queue__jki_lib_state_machine.vi"("State(s) in Front (\"\")"="File: Save", "State(s) in (\"\")"=w82) -> ("States Out"=w81:string)  [unwired: 13 in]
          }
          event "PROCESS": Value Change {
            n36 = event-data() -> ()  [unwired: 1 in, 6 out]
            n37 = local write "PROCESS"(FALSE ("PROCESS")) -> ()
            n38 = call <vilib>:"Add State(s) to Queue__jki_lib_state_machine.vi"("State(s) in Front (\"\")"="Macro: Process" ("State(s) in Front (\"\")"), "State(s) in (\"\")"=w88) -> ("States Out"=w87:string)  [unwired: 13 in]
          }
          event "CLEAR": Value Change {
            n39 = event-data() -> ()  [unwired: 1 in, 6 out]
            n40 = local write "CLEAR"(FALSE ("CLEAR")) -> ()
            n41 = local write "Process Queue"("" ("Process States")) -> ()
            n42 = call <vilib>:"Add State(s) to Queue__jki_lib_state_machine.vi"("State(s) in (\"\")"=w94) -> ("States Out"=w93:string)  [unwired: 14 in]
          }
          event Panel Close? {
            # "Discard the event because we'll close the front panel ourselves in Macro: Exit"
            # "Close Panel button (pressed) Event\n(this executes Macro: Exit to terminate the VI)"
            n43 = event-data() -> ()  [unwired: 1 in, 1 out]
            n44 = event-data("Discard?"=TRUE) -> ()  [unwired: 1 in, 1 out]
            n45 = call <vilib>:"Add State(s) to Queue__jki_lib_state_machine.vi"("State(s) in Front (\"\")"="Macro: Exit", "State(s) in (\"\")"=w100) -> ("States Out"=w99:string)  [unwired: 13 in]
          }
        }
      }
      frame "---------- Core ----------" {
        # "Do not put any code in this frame.\n(it is a separator no-op)"
        n46 = call <vilib>:"Add State(s) to Queue__jki_lib_state_machine.vi"("State(s) in (\"\")"=w104) -> ("States Out"=w103:string)  [unwired: 14 in]
      }
      frame Default {
        w114 = 42 items=["No error", "Argument error", "Memory is full", "Out of zone", "End of file", "File already open", "Generic file I/O error", "File not found", "File permission error", "Disk is full", "Duplicate path", "Too many files open", "System feature not enabled", "Resource file not found", "Cannot add resource", "Resource not found", "Image not found", "Image memory error", "Pen does not exist", "Config type invalid", "Config token not found", "Config parse error", "Config memory error", "Bad external code format", "Bad external code offset", "External code not present", "Null window", "Destroy window error", "Null menu", "Print aborted", "Bad print record", "Print driver error", "Windows error during printing", "Memory error during printing", "Print dialog error", "Generic print error", "Invalid device refnum", "Device not found", "Device parameter error", "Device unit error", "Cannot open device", "Device call aborted", "Generic error", "Cancelled by user", "Object ID too low", "Object ID too high", "Object not in heap", "Unknown heap", "Unknown object (invalid DefProc)", "Unknown object (DefProc not in table)", "Message out of range", "Invalid (null) method", "Unknown message", "Manager call not supported", "Bad address", "Network operation in progress", "Network operation timed out", "Connection is busy", "Network attribute not supported", "Network error", "Address in use", "System out of memory", "Connection aborted", "Connection refused", "Not connected", "Already connected", "Connection closed", "Initialization error (interapplication manager)", "Bad occurrence", "Wait on unbound occurrence handler", "Occurrence queue overflow", "Datalog type conflict", "Unused", "Unrecognized type (interapplication manager)", "Memory corrupt", "Failed to make temporary DLL", "Old CIN version", "Drag socket not found", "Failed to load drop-object", "Failed to register OLE object", "Failed to release OLE object", "Format specifier type mismatch", "Unknown format specifier", "Too few format specifiers", "Too many format specifiers", "Scan failed", "Newer CIN version", "Error converting to variant", "Runtime menu error", "Password tampered", "Variant attribute not found", "Incompatible variant data type", "Event data is not available", "Event Store is not present", "Occurrence is not found", "Event Queue is not created", "Event info is not available", "Refnum passed is NULL", "Error retrieving Class GUID", "Error retrieving CoClass GUID", "Error retrieving TypeLib GUID.", "Bad built application magic bytes.", "Specific driver is different from the specific driver associated with the Logical Name.", "There is no session opened to the class driver.", "Max Error", "MAX - Error with config objects", "MAX - Error loading configuration", "MAX - Group not supported"]
        # "Current State"
        # "Do not delete, rename, or modify this frame.\n(this is used to capture unhandled states and typos)"
        # "Handle mistyped state name (developer tool)"
        n47 = Format Into String(format string="Software Exception: Unhandled State \"%s\"." ("message"), error in=w110, w105) -> (resulting string=w113:string, error out=w112:errorcluster)  [unwired: 1 in]
        n48 = call <vilib>:"Error Cluster From Error Code.vi"("show call chain? (False)"=TRUE, "error in (no error)"=w112, "error message (\"\")"=w113, "error code (0)"=w114) -> ("error out"=w111:errorcluster)  [unwired: 5 in]
        n49 = call <vilib>:"Add State(s) to Queue__jki_lib_state_machine.vi"("State(s) in (\"\")"=w109) -> ("States Out"=w108:string)  [unwired: 14 in]
      }
      frame "Initialize Core Data" {
        # "Do not delete, rename, or modify this frame.\n(this is used to determine panel behavior on exit)"
        # "originally closed?"
        # "exe?"
        # "If panel starts closed or is an EXE, then close it when we exit"
        n50 = property class="VI"() -> ("FP.State"=w118:T4)  [unwired: 2 in, 2 out]
        n51 = property class="App"() -> ("App.Kind"=w124:T5)  [unwired: 2 in, 2 out]
        n52 = control-ref of="Current VI Reference"() -> (w119:refnum<vi>)
        n53 = Equal?(x=w118, y=T4."Closed" ("Front Panel Window:State")) -> (x = y?=w116:bool)
        n54 = Equal?(x=w124, y=T5."Run Time System" ("Application:Kind")) -> (x = y?=w122:bool)
        n55 = Or(x=w116, y=w122) -> (x .or. y?=w120:bool)
        n56 = Bundle By Name(cluster=w121, "Core.Current VI Reference"=w119, "Core.Close Panel on Exit?"=w120) -> (w126:T7)
        n57 = call <vilib>:"Add State(s) to Queue__jki_lib_state_machine.vi"("State(s) in (\"\")"=w128) -> ("States Out"=w127:string)  [unwired: 14 in]
      }
      frame "Error Handler" {
        # "Unhandled Error -- Display it"
        # "Handle any errors here.\nYou can also output any states to clean-up after errors occur"
        # "Clear error"
        n58 = call <vilib>:"General Error Handler.vi"("error in (no error)"=w130) -> ()  [unwired: 10 in, 5 out]
        n59 = call <vilib>:"Add State(s) to Queue__jki_lib_state_machine.vi"("State(s) in Front (\"\")"="/* Post Error States", "State(s) in (\"\")"=w134) -> ("States Out"=w133:string)  [unwired: 13 in]
      }
      frame "Exit" {
        # "Do not put any code in this frame.\n(No errors that occur here will be handled.)"
        n60 = call <vilib>:"Add State(s) to Queue__jki_lib_state_machine.vi"("State(s) in (\"\")"=w139) -> ("States Out"=w138:string)  [unwired: 14 in]
      }
      frame "---------- Data ----------" {
        # "Do not put any code in this frame.\n(It is a separator no-op. You can make a copy of this frame to create a new Data frame)"
        n61 = call <vilib>:"Add State(s) to Queue__jki_lib_state_machine.vi"("State(s) in (\"\")"=w143) -> ("States Out"=w142:string)  [unwired: 14 in]
      }
      frame "Data: Initialize" {
        w144 = path[] []  # Paths
        w145 = T9 {"X"="", "Y"="", "Z"="", "A"="", "B"="", "C"=""}  # Keys
        w146 = cluster{"Data (Dictionary)":T6[]}[] []  # Dictionaries
        w148 = cluster{"X-array":dbl[], "Y-array":dbl[]}[] []  # XY Data (processed 2)
        w147 = cluster{"X-array":dbl[], "Y-array":dbl[]}[] []  # XY Data (processed 1)
        w149 = cluster{"X-array":dbl[], "Y-array":dbl[]}[] []  # XY Data (unprocessed)
        w150 = T10 {"X"=refnum, "Y"=refnum, "Z"=refnum, "A"=refnum, "B"=refnum, "C"=refnum}  # Rings
        w151 = path ""  # Path
        w152 = T11 {"Data: Unprocessed"=refnum, "Data: Processed"=refnum, "Data: Intensity/Vertical"=refnum, "Data: Intensity/Horizontal"=refnum, "Differential: Intensity/Vertical"=refnum, "Differential: Intensity/Horizontal"=refnum}  # Graph
        w153 = dbl[] []  # Parameter
        w154 = T12 {"Current VI Reference"=refnum, "Close Panel on Exit?"=FALSE}  # Core
        # "do not delete - used by framework"
        # "Initialize the shift-register data, here.\n(data names are defined by what you wire into the bundle function)"
        n62 = Bundle("Core"=w154, "Path"=w151, "Paths"=w144, "Graph"=w152, "Rings"=w150, "Dictionaries"=w146, "Keys"=w145, "XY Data (unprocessed)"=w149, "XY Data (processed 1)"=w147, "XY Data (processed 2)"=w148, "Parameter"=w153) -> (w156:T7)  [unwired: 1 in]
        n63 = call <vilib>:"Add State(s) to Queue__jki_lib_state_machine.vi"("State(s) in (\"\")"=w158) -> ("States Out"=w157:string)  [unwired: 14 in]
      }
      frame "Data: Get Keys" {
        # "Do not put any code in this frame.\n(It is a separator no-op. You can make a copy of this frame to create a new Macro frame)"
        n64 = Unbundle By Name(w166) -> ("Keys"=w163:T9, "Rings"=w171:T10)
        n65 = Cluster To Array(cluster=w171) -> (array=w170:refnum<vi>[])
        n66 = for {
          tunnel: w170 -> [w177] mode=indexing
          tunnel: w168 -> [w176]
          tunnel: [w175] -> w169 mode=indexing
          tunnel: [w174] -> w165 mode=indexing
          n67 = property class="Ring (strict)"(reference=w177, error in=w176) -> (error out=w175:errorcluster, "RingText.Text"=w174:string)  [unwired: 1 out]
        }
        n68 = Merge Errors(w169) -> (w159:errorcluster)
        n69 = call <userlib>:"Array to VCluster__ogtk.vi"("error in (no error)"=w159, "Array"=w165) -> ("error out"=w161:errorcluster, "VCluster"=w164:variant)  [unwired: 8 in]
        n70 = Variant To Data(error in=w161, type=w163, Variant=w164) -> (data=w162:T9, error out=w160:errorcluster)
        n71 = Bundle By Name(cluster=w166, "Keys"=w162) -> (w167:T7)
        n72 = call <vilib>:"Add State(s) to Queue__jki_lib_state_machine.vi"("State(s) in (\"\")"=w173) -> ("States Out"=w172:string)  [unwired: 14 in]
      }
      frame "Data: Select Channels" {
        # "Do not put any code in this frame.\n(It is a separator no-op. You can make a copy of this frame to create a new Data frame)"
        n73 = Unbundle By Name(w187) -> ("Parameter"=w180:dbl[], "Dictionaries"=w182:cluster{"Data (Dictionary)":T6[]}[], "Keys"=w189:T9)
        n74 = for {
          tunnel: w189 -> [w208]
          tunnel: [w207] -> w185
          tunnel: [w206] -> w184 mode=indexing
          tunnel: [w205] -> w181 mode=indexing
          tunnel: w182 -> [w203] mode=indexing
          # "C"
          # "B"
          # "A"
          # "Z"
          # "Y"
          # "X"
          n75 = Unbundle(w203) -> ("Data (Dictionary)"=w204:T6[])
          n76 = Unbundle By Name(w208) -> ("X"=w194:string)  [unwired: 5 out]
          n77 = Cluster To Array(cluster=w208) -> (array=w192:string[])
          n78 = for {
            tunnel: w204 -> [w212]
            tunnel: w192 -> [w211] mode=indexing
            tunnel: [w210] -> w201 mode=indexing
            tunnel: [w209] -> w200 mode=indexing
            n79 = call "Get Map Value.vim"("Key"=w211, "map in"=w212) -> ("error out"=w213:errorcluster, "value"=w214:variant)  [unwired: 7 in, 1 out]
            n80 = call <userlib>:"Variant to DBL Array.vi"("error in (no error)"=w213, "Data (Variant)"=w214) -> ("error out"=w210:errorcluster, "1D Array"=w209:dbl[])  [unwired: 7 in, 1 out]
          }
          n81 = disable-structure shown="Disabled" {
            disable-tunnel: w204 -> [w219 _]
            disable-tunnel: [w218 _] -> _
            disable-tunnel: [w217 _] -> _
            disable-tunnel: [w216 _] -> _
            disable-tunnel: w194 -> [w215 _]
            frame Disabled {
              # "parse the dictionary"
              n82 = call "Convert Dictionary to Map.vim"("Data (Dictionary)"=w219) -> ("map out"=w220:T13)  [unwired: 9 in, 1 out]
              n83 = call "Get Map Value.vim"("Key"=w215, "map in"=w219) -> ("value"=w218:variant)  [unwired: 7 in, 2 out]
              n84 = call "Get Map Value.vim"("Key"=w215, "map in"=w220) -> ("value"=w217:variant)  [unwired: 7 in, 2 out]
              n85 = Look In Map(map=w220, key=w215) -> (value=w216:variant)  [unwired: 1 in, 1 out]
            }
            frame Enabled {
            }
          }
          n86 = Index Array(array=w200) -> (element #1=w196:dbl[], element #2=w195:dbl[], element #4=w193:dbl[], element #5=w199:dbl[], element #6=w198:dbl[])  [unwired: 12 in, 1 out]
          n87 = Subtract(x=w199, y=w198) -> (x-y=w197:dbl[])
          n88 = Divide(x=w193, y=w197) -> (x/y=w202:dbl[])
          n89 = Merge Errors(w201) -> (w207:errorcluster)
          n90 = Reciprocal(x=w202) -> ()  [unwired: 1 out]
          n91 = call-poly <vilib>:"Mean.vi"("X"=w195) -> ("mean"=w205:dbl)  [unwired: 1 out]
          n92 = Bundle("1D Array"=w196, "1D Array"=w193) -> (w206:cluster{"1D Array":dbl[], "1D Array":dbl[]})  [unwired: 1 in]
        }
        n93 = local read "param in notes"() -> (w179:bool)
        n94 = Select(t=w180, s=w179, f=w181) -> (s? t:f=w178:dbl[])
        n95 = Bundle By Name(cluster=w187, "Parameter"=w178, "XY Data (unprocessed)"=w184, "XY Data (processed 1)"=w184, "XY Data (processed 2)"=w184) -> (w188:T7)
        n96 = Merge Errors(w185, w183) -> (w186:errorcluster)
        n97 = call <vilib>:"Add State(s) to Queue__jki_lib_state_machine.vi"("State(s) in (\"\")"=w191) -> ("States Out"=w190:string)  [unwired: 14 in]
      }
      frame "Data: Cleanup" {
        # "Cleanup any data and references, here.\n(this is called automatically, by the Macro: Exit)"
        n98 = Unbundle By Name(w221) -> ("Core.Current VI Reference"=w224:refnum<vi>)
        n99 = Close Reference(reference=w224, error in (no error)=w223) -> (error out=w222:errorcluster)
        n100 = call <vilib>:"Add State(s) to Queue__jki_lib_state_machine.vi"("State(s) in (\"\")"=w226) -> ("States Out"=w225:string)  [unwired: 14 in]
      }
      frame "---------- UI ----------" {
        # "Do not put any code in this frame.\n(It is a separator no-op. You can make a copy of this frame to create a new UI frame)"
        n101 = call <vilib>:"Add State(s) to Queue__jki_lib_state_machine.vi"("State(s) in (\"\")"=w230) -> ("States Out"=w229:string)  [unwired: 14 in]
      }
      frame "UI: Initialize" {
        w236 = "" ("Process States")
        # "Initialize the User Interface, here.\n(this is called automatically, by the Macro: Init)"
        n102 = property on="Available States" class="LstBox (strict)"("Val(Sgnl)"=-1 ("Value (Signaling)"), "Item Names"=string[] ["XY: Add", "XY: Subtract", "XY: Multiply", "XY: Divide", "XY: Square", "XY: Log", "XY: Sort", "XY: Swap", "XY: Reverse", "XY: Subset", "XY: Derivative", "XY: Difference Quotient", "XY: Interpolate", "XY: Decimate", "XY: Average", "XY: Moving Average", "XY: SG Filter", "XY: Zero Phase Filter", "XY: Symmeterize", "XY: FFT Spectrum", "XY: FFT Power Spectrum"]) -> ()  [unwired: 2 in, 2 out]
        n103 = local write "Graphs Tab Control"(enum32{"Data", "Intensity/Linecuts"}."Data" ("Graphs Tab Control")) -> ()
        n104 = local write "Tab Control"(enum32{"Load Data"}."Load Data" ("Tab Control")) -> ()
        n105 = local write "Processed States"(w236) -> ()
        n106 = property on="Path" class="Path"("Val(Sgnl)"="Path") -> ()  [unwired: 2 in, 2 out]
        n107 = local write "Process Queue"(w236) -> ()
        n108 = call <userlib>:"Fit VI window to Content__ogtk.vi"("error in (no error)"=w234, "border spacing (2 px)"=0) -> ("error out"=w233:errorcluster)  [unwired: 4 in, 1 out]
        n109 = call <vilib>:"Add State(s) to Queue__jki_lib_state_machine.vi"("State(s) in (\"\")"=w242) -> ("States Out"=w241:string)  [unwired: 14 in]
      }
      frame "UI: Cursor Set" {
        # "Argument"
        # "Set and Unset Cursor Busy.\n(Usage: \"UI: Cursor Set >> Busy|Idle\")"
        n110 = case shown="\"Idle\", Default" w243 {
          tunnel: w245 -> [w250 w252]
          tunnel: [w249 w251] -> w244
          frame "Idle", Default {
            n111 = call <vilib>:"Unset Busy.vi"("error in (no error)"=w250) -> ("error out"=w249:errorcluster)  [unwired: 10 in]
          }
          frame "Busy" {
            n112 = call <vilib>:"Set Busy.vi"("error in (no error)"=w252) -> ("error out"=w251:errorcluster)  [unwired: 9 in, 1 out]
          }
        }
        n113 = call <vilib>:"Add State(s) to Queue__jki_lib_state_machine.vi"("State(s) in (\"\")"=w248) -> ("States Out"=w247:string)  [unwired: 14 in]
      }
      frame "UI: Front Panel State" {
        # "Argument"
        # "Set Front Panel Open or Closed\n(Usage: \"UI: Front Panel State >> Open|Close\")"
        n114 = Unbundle By Name(w255) -> ("Core.Current VI Reference"=w254:refnum<vi>)
        n115 = case shown="\"Maximize\", \"Maximized\"" w253 {
          tunnel: w257 -> [w265 w280 w291 w304 w317]
          tunnel: [w267 w281 w293 w306 w319] -> w256
          tunnel: w254 -> [w266 w278 w292 w305 w318]
          frame "Open", "Standard", Default {
            w260 = T4."Standard" ("State")
            n116 = property class="VI"(reference=w266, error in=w265) -> (reference out=w263:refnum<vi>, error out=w264:errorcluster, "FP.State"=w262:T4)
            n117 = Not Equal?(x=w262, y=w260) -> (x != y?=w261:bool)
            n118 = case shown="True" w261 {
              tunnel: [w271 w273] -> w267
              tunnel: w264 -> [w270 w273]
              tunnel: w263 -> [w269 _]
              tunnel: w260 -> [w268 _]
              frame True {
                n119 = invoke class="VI" method="FP.Open"(reference=w269, error in=w270, "Activate"=TRUE, "State"=w268) -> (error out=w271:errorcluster)  [unwired: 1 in, 4 out]
              }
              frame False {
              }
            }
          }
          frame "Close", "Closed" {
            n120 = property class="VI"(reference=w278, error in=w280) -> (reference out=w277:refnum<vi>, error out=w279:errorcluster, "FP.State"=w275:T4)
            n121 = Not Equal?(x=w275, y=T4."Closed" ("Front Panel Window:State")) -> (x != y?=w274:bool)
            n122 = case shown="True" w274 {
              tunnel: [w282 w285] -> w281
              tunnel: w279 -> [w282 w284]
              tunnel: w277 -> [_ w283]
              frame False {
              }
              frame True {
                n123 = invoke class="VI" method="FP.Close"(reference=w283, error in=w284) -> (error out=w285:errorcluster)  [unwired: 1 in, 2 out]
              }
            }
          }
          frame "Hidden", "Hide" {
            w286 = T4."Hidden" ("State")
            n124 = property class="VI"(reference=w292, error in=w291) -> (reference out=w289:refnum<vi>, error out=w290:errorcluster, "FP.State"=w288:T4)
            n125 = Not Equal?(x=w288, y=w286) -> (x != y?=w287:bool)
            n126 = case shown="True" w287 {
              tunnel: [w297 w298] -> w293
              tunnel: w290 -> [w296 w298]
              tunnel: w289 -> [w295 _]
              tunnel: w286 -> [w294 _]
              frame True {
                n127 = invoke class="VI" method="FP.Open"(reference=w295, error in=w296, "State"=w294) -> (error out=w297:errorcluster)  [unwired: 2 in, 4 out]
              }
              frame False {
              }
            }
          }
          frame "Minimize", "Minimized" {
            w299 = T4."Minimized" ("State")
            n128 = property class="VI"(reference=w305, error in=w304) -> (reference out=w302:refnum<vi>, error out=w303:errorcluster, "FP.State"=w301:T4)
            n129 = Not Equal?(x=w301, y=w299) -> (x != y?=w300:bool)
            n130 = case shown="True" w300 {
              tunnel: [w310 w311] -> w306
              tunnel: w303 -> [w309 w311]
              tunnel: w302 -> [w308 _]
              tunnel: w299 -> [w307 _]
              frame True {
                n131 = invoke class="VI" method="FP.Open"(reference=w308, error in=w309, "State"=w307) -> (error out=w310:errorcluster)  [unwired: 2 in, 4 out]
              }
              frame False {
              }
            }
          }
          frame "Maximize", "Maximized" {
            w312 = T4."Maximized" ("State")
            n132 = property class="VI"(reference=w318, error in=w317) -> (reference out=w315:refnum<vi>, error out=w316:errorcluster, "FP.State"=w314:T4)
            n133 = Not Equal?(x=w314, y=w312) -> (x != y?=w313:bool)
            n134 = case shown="True" w313 {
              tunnel: [w323 w324] -> w319
              tunnel: w316 -> [w322 w324]
              tunnel: w315 -> [w321 _]
              tunnel: w312 -> [w320 _]
              frame True {
                n135 = invoke class="VI" method="FP.Open"(reference=w321, error in=w322, "State"=w320) -> (error out=w323:errorcluster)  [unwired: 2 in, 4 out]
              }
              frame False {
              }
            }
          }
        }
        n136 = call <vilib>:"Add State(s) to Queue__jki_lib_state_machine.vi"("State(s) in (\"\")"=w259) -> ("States Out"=w258:string)  [unwired: 14 in]
      }
      frame "---------- Macro ----------" {
        # "Do not put any code in this frame.\n(It is a separator no-op. You can make a copy of this frame to create a new Macro frame)"
        n137 = call <vilib>:"Add State(s) to Queue__jki_lib_state_machine.vi"("State(s) in (\"\")"=w328) -> ("States Out"=w327:string)  [unwired: 14 in]
      }
      frame "Macro: Initialize" {
        # "Initialization Macro\n(This is called once, when the VI starts)"
        n138 = call <vilib>:"Add State(s) to Queue__jki_lib_state_machine.vi"("State(s) in Front (\"\")"="Data: Initialize\nInitialize Core Data\nUI: Initialize\nUI: Front Panel State >> Open\nGraph: Initialize References 1\nGraph: Initialize References 2\nGraph: Initialize References 3\nGraph: Update Color 1\nGraph: Update Color 2", "State(s) in (\"\")"=w333) -> ("States Out"=w332:string)  [unwired: 13 in]
      }
      frame "Macro: Exit" {
        # "Exit Macro\n(This is called once, when the VI exits)"
        n139 = Unbundle By Name(w340) -> ("Core.Close Panel on Exit?"=w339:bool)
        n140 = Select(t="UI: Front Panel State >> Close", s=w339, f="") -> (s? t:f=w336:string)
        n141 = call <vilib>:"Add State(s) to Queue__jki_lib_state_machine.vi"("State(s) in (\"\")"=w336, "State(s) at Back (\"\")"="Graph: Clear\nData: Cleanup\nExit") -> ("States Out"=w334:string)  [unwired: 13 in]
        n142 = call <vilib>:"Add State(s) to Queue__jki_lib_state_machine.vi"("State(s) in Front (\"\")"=w334, "State(s) in (\"\")"=w343) -> ("States Out"=w342:string)  [unwired: 13 in]
      }
      frame "Macro: Process" {
        # "XY: Add\nXY: Subtract\nXY: Multiply\nXY: Divide\nXY: Sort\nXY: Swap\nXY: Reverse\nXY: Subset\nXY: Derivative\nXY: Interpolate\nXY: FFT Spectrum\nXY: FFT Power Spectrum"
        # "Do not put any code in this frame.\n(It is a separator no-op. You can make a copy of this frame to create a new Macro frame)"
        n143 = Format Into String(format string="UI: Cursor Set >> Busy\nFile: List Folder\nFile: Load\nData: Get Keys\nData: Select Channels\nGraph: Initialize Graphs\nXY: Subset >>%s" ("State(s) in Front (\"\")"), enum16{"Slider (%)", "X[] min and max"}."X[] min and max" ("Method")) -> (resulting string=w345:string)  [unwired: 2 in, 1 out]
        n144 = call <vilib>:"Add State(s) to Queue__jki_lib_state_machine.vi"("State(s) in Front (\"\")"=w345, "State(s) in (\"\")"="Process Queue", "State(s) at Back (\"\")"="Graph: Update Graphs\nUI: Cursor Set >> Idle" ("State(s) in Front (\"\")")) -> ("States Out"=w348:string)  [unwired: 12 in]
        "Processed States" <- w348
        n145 = call <vilib>:"Add State(s) to Queue__jki_lib_state_machine.vi"("State(s) in Front (\"\")"=w348, "State(s) in (\"\")"=w353) -> ("States Out"=w352:string)  [unwired: 13 in]
      }
      frame "---------- Graph ----------" {
        # "Do not put any code in this frame.\n(It is a separator no-op. You can make a copy of this frame to create a new Macro frame)"
        n146 = call <vilib>:"Add State(s) to Queue__jki_lib_state_machine.vi"("State(s) in (\"\")"=w357) -> ("States Out"=w356:string)  [unwired: 14 in]
      }
      frame "Graph: Controls" {
        # "Do not put any code in this frame.\n(It is a separator no-op. You can make a copy of this frame to create a new Macro frame)"
        n147 = call <vilib>:"Add State(s) to Queue__jki_lib_state_machine.vi"("State(s) in (\"\")"=w361) -> ("States Out"=w360:string)  [unwired: 14 in]
      }
      frame "Graph: Initialize References 1" {
        # "Do not put any code in this frame.\n(It is a separator no-op. You can make a copy of this frame to create a new Data frame)"
        n148 = control-ref of="XY Graph: Unprocessed"() -> (w372:refnum<vi>)
        n149 = control-ref of="Data Intensity"() -> (w367:refnum<vi>)
        n150 = control-ref of="XY Graph: Processed"() -> (w366:refnum<vi>)
        n151 = call <vilib>:"Write Intensity Graph ref.vi"("error in (no error)"=w365, "Intensity Graph"=w367) -> ("error out"=w373:errorcluster, "graph_utilities out"=w371:refnum<class "graph_utilities.lvclass">)  [unwired: 8 in]
        n152 = call <vilib>:"Write Intensity Graph ref.vi"("error in (no error)"=w365, "Intensity Graph"=w367) -> ("error out"=w368:errorcluster, "graph_utilities out"=w363:refnum<class "graph_utilities.lvclass">)  [unwired: 8 in]
        n153 = call <vilib>:"Write XY Graph ref.vi"("error in (no error)"=w373, "XY Graph"=w372, "graph_utilities in"=w371) -> ("error out"=w369:errorcluster, "graph_utilities out"=w370:refnum<class "graph_utilities.lvclass">)  [unwired: 7 in]
        n154 = call <vilib>:"Write XY Graph ref.vi"("error in (no error)"=w368, "XY Graph"=w366, "graph_utilities in"=w363) -> ("error out"=w364:errorcluster, "graph_utilities out"=w362:refnum<class "graph_utilities.lvclass">)  [unwired: 7 in]
        n155 = Bundle By Name(cluster=w376, "Graph.Data: Unprocessed"=w370, "Graph.Data: Processed"=w362) -> (w375:T7)
        n156 = Merge Errors(w369, w364) -> (w374:errorcluster)
        n157 = call <vilib>:"Add State(s) to Queue__jki_lib_state_machine.vi"("State(s) in (\"\")"=w378) -> ("States Out"=w377:string)  [unwired: 14 in]
      }
      frame "Graph: Initialize References 2" {
        # "Do not put any code in this frame.\n(It is a separator no-op. You can make a copy of this frame to create a new Data frame)"
        n158 = control-ref of="Data Vertical"() -> (w398:refnum<vi>)
        n159 = control-ref of="Data Horizontal"() -> (w392:refnum<vi>)
        n160 = control-ref of="Diff Vertical"() -> (w397:refnum<vi>)
        n161 = control-ref of="Diff Horizontal"() -> (w395:refnum<vi>)
        n162 = control-ref of="Data Intensity"() -> (w380:refnum<vi>)
        n163 = control-ref of="Diff Intensity"() -> (w390:refnum<vi>)
        n164 = call <vilib>:"Write Intensity Graph ref.vi"("error in (no error)"=w379, "Intensity Graph (Control)"=w380, "Intensity Graph"=w380) -> ("error out"=w391:errorcluster, "graph_utilities out"=w393:refnum<class "graph_utilities.lvclass">)  [unwired: 7 in]
        n165 = call <vilib>:"Write Intensity Graph ref.vi"("error in (no error)"=w379, "Intensity Graph (Control)"=w380, "Intensity Graph"=w390) -> ("error out"=w394:errorcluster, "graph_utilities out"=w396:refnum<class "graph_utilities.lvclass">)  [unwired: 7 in]
        n166 = call <vilib>:"Write XY Graph ref.vi"("error in (no error)"=w391, "XY Graph"=w392, "graph_utilities in"=w393) -> ("error out"=w388:errorcluster, "graph_utilities out"=w383:refnum<class "graph_utilities.lvclass">)  [unwired: 7 in]
        n167 = call <vilib>:"Write XY Graph ref.vi"("error in (no error)"=w394, "XY Graph"=w395, "graph_utilities in"=w396) -> ("error out"=w389:errorcluster, "graph_utilities out"=w381:refnum<class "graph_utilities.lvclass">)  [unwired: 7 in]
        n168 = call <vilib>:"Write XY Graph ref.vi"("error in (no error)"=w388, "XY Graph"=w398, "graph_utilities in"=w393) -> ("error out"=w387:errorcluster, "graph_utilities out"=w384:refnum<class "graph_utilities.lvclass">)  [unwired: 7 in]
        n169 = call <vilib>:"Write XY Graph ref.vi"("error in (no error)"=w389, "XY Graph"=w397, "graph_utilities in"=w396) -> ("error out"=w386:errorcluster, "graph_utilities out"=w382:refnum<class "graph_utilities.lvclass">)  [unwired: 7 in]
        n170 = Bundle By Name(cluster=w400, "Graph.Data: Intensity/Vertical"=w384, "Graph.Data: Intensity/Horizontal"=w383, "Graph.Differential: Intensity/Vertical"=w382, "Graph.Differential: Intensity/Horizontal"=w381) -> (w399:T7)
        n171 = Merge Errors(w387, w386) -> (w385:errorcluster)
        n172 = call <vilib>:"Add State(s) to Queue__jki_lib_state_machine.vi"("State(s) in (\"\")"=w402) -> ("States Out"=w401:string)  [unwired: 14 in]
      }
      frame "Graph: Initialize References 3" {
        # "Do not put any code in this frame.\n(It is a separator no-op. You can make a copy of this frame to create a new Macro frame)"
        n173 = control-ref of="X"() -> (w403:refnum<vi>)
        n174 = control-ref of="Y"() -> (w404:refnum<vi>)
        n175 = control-ref of="Z"() -> (w405:refnum<vi>)
        n176 = control-ref of="A"() -> (w406:refnum<vi>)
        n177 = control-ref of="B"() -> (w407:refnum<vi>)
        n178 = control-ref of="C"() -> (w408:refnum<vi>)
        n179 = Bundle By Name(cluster=w409, "Rings.X"=w403, "Rings.Y"=w404, "Rings.Z"=w405, "Rings.A"=w406, "Rings.B"=w407, "Rings.C"=w408) -> (w410:T7)
        n180 = call <vilib>:"Add State(s) to Queue__jki_lib_state_machine.vi"("State(s) in (\"\")"=w413) -> ("States Out"=w412:string)  [unwired: 14 in]
      }
      frame "Graph: Initialize Graphs" {
        # "Do not put any code in this frame.\n(It is a separator no-op. You can make a copy of this frame to create a new Macro frame)"
        n181 = Unbundle By Name(w420) -> ("Graph.Data: Unprocessed"=w421:refnum<class "graph_utilities.lvclass">, "XY Data (unprocessed)"=w417:cluster{"X-array":dbl[], "Y-array":dbl[]}[], "Parameter"=w414:dbl[])
        n182 = disable-structure shown="Enabled" {
          disable-tunnel: w421 -> [w433 w435]
          disable-tunnel: w419 -> [w432 _]
          disable-tunnel: w417 -> [w431 w434]
          disable-tunnel: [w430 _] -> w416
          disable-tunnel: [w429 w435] -> w415
          disable-tunnel: [_ w434] -> _
          frame Enabled {
            n183 = call-poly <vilib>:"Set XY Graph Value.vi"("error in (no error)"=w432, "XY-data"=w431, "graph_utilities in"=w433) -> ("error out"=w430:errorcluster, "graph_utilities out"=w429:refnum<class "graph_utilities.lvclass">)  [unwired: 7 in]
          }
          frame Disabled {
            # "This preferred over Set XY Graph Value"
            "XY Graph: Unprocessed" <- w434
          }
        }
        n184 = disable-structure shown="Enabled" {
          disable-tunnel: [w427 w428] -> w418
          disable-tunnel: w416 -> [w426 w428]
          disable-tunnel: w415 -> [w425 _]
          disable-tunnel: w414 -> [w424 _]
          frame Disabled {
            n185 = call <vilib>:"XY Graph to Intensity Graph.vi"("error in (no error)"=w426, "Y Scale"=w424, "graph_utilities in"=w425) -> ("error out"=w427:errorcluster)  [unwired: 7 in, 1 out]
          }
          frame Enabled {
          }
        }
        n186 = call <vilib>:"Add State(s) to Queue__jki_lib_state_machine.vi"("State(s) in (\"\")"=w423) -> ("States Out"=w422:string)  [unwired: 14 in]
      }
      frame "Graph: Update Graphs" {
        # "Do not put any code in this frame.\n(It is a separator no-op. You can make a copy of this frame to create a new UI frame)"
        n187 = Unbundle By Name(w448) -> ("Graph.Data: Processed"=w447:refnum<class "graph_utilities.lvclass">, "XY Data (processed 1)"=w446:cluster{"X-array":dbl[], "Y-array":dbl[]}[], "Parameter"=w436:dbl[])
        n188 = flat-sequence {
          tunnel: [w452] -> w438
          tunnel: [w451] -> w442
          tunnel: w443 -> [w451]
          frame #0 {
            n189 = call <vilib>:"High Resolution Relative Seconds.vi"() -> ("relative seconds"=w452:dbl)
          }
        }
        n190 = disable-structure shown="Enabled" {
          disable-tunnel: w447 -> [w459 w461]
          disable-tunnel: w446 -> [w458 w460]
          disable-tunnel: [w457 w461] -> w445
          disable-tunnel: [w456 _] -> w444
          disable-tunnel: w442 -> [w455 _]
          disable-tunnel: [_ w460] -> _
          frame Enabled {
            n191 = call-poly <vilib>:"Set XY Graph Value.vi"("error in (no error)"=w455, "XY-data"=w458, "graph_utilities in"=w459) -> ("error out"=w456:errorcluster, "graph_utilities out"=w457:refnum<class "graph_utilities.lvclass">)  [unwired: 7 in]
          }
          frame Disabled {
            # "This preferred over Set XY Graph Value"
            "XY Graph: Processed" <- w460
          }
        }
        n192 = call <vilib>:"XY Graph to Intensity Graph.vi"("error in (no error)"=w444, "Y Scale"=w436, "graph_utilities in"=w445) -> ("error out"=w441:errorcluster)  [unwired: 7 in, 1 out]
        n193 = flat-sequence {
          tunnel: [w454] -> w439
          tunnel: [w453] -> w440
          tunnel: w441 -> [w453]
          frame #0 {
            n194 = call <vilib>:"High Resolution Relative Seconds.vi"() -> ("relative seconds"=w454:dbl)
          }
        }
        n195 = Subtract(x=w439, y=w438) -> (x-y=→"time (ms)":dbl)
        n196 = call <vilib>:"Add State(s) to Queue__jki_lib_state_machine.vi"("State(s) in (\"\")"=w450) -> ("States Out"=w449:string)  [unwired: 14 in]
      }
      frame "Graph: Clear" {
        w462 = cluster{dbl[], dbl[]}[] [] ("Value")
        w465 = dbl[][] [] ("Value")
        # "Do not put any code in this frame.\n(It is a separator no-op. You can make a copy of this frame to create a new Macro frame)"
        n197 = Unbundle By Name(w482) -> ("Graph.Data: Unprocessed"=w466:refnum<class "graph_utilities.lvclass">, "Graph.Data: Processed"=w481:refnum<class "graph_utilities.lvclass">, "Graph.Data: Intensity/Vertical"=w475:refnum<class "graph_utilities.lvclass">, "Graph.Data: Intensity/Horizontal"=w474:refnum<class "graph_utilities.lvclass">, "Graph.Differential: Intensity/Vertical"=w473:refnum<class "graph_utilities.lvclass">, "Graph.Differential: Intensity/Horizontal"=w472:refnum<class "graph_utilities.lvclass">)
        n198 = call <vilib>:"Set Intensity Graph Value.vi"("Value"=w465, "graph_utilities in"=w466) -> ("error out"=w463:errorcluster, "graph_utilities out"=w464:refnum<class "graph_utilities.lvclass">)  [unwired: 8 in]
        n199 = call <vilib>:"Set Intensity Graph Value.vi"("Value"=w465, "graph_utilities in"=w481) -> ("error out"=w471:errorcluster, "graph_utilities out"=w480:refnum<class "graph_utilities.lvclass">)  [unwired: 8 in]
        n200 = call <vilib>:"Set Intensity Graph Value.vi"("Value"=w465, "graph_utilities in"=w474) -> ("error out"=w469:errorcluster, "graph_utilities out"=w478:refnum<class "graph_utilities.lvclass">)  [unwired: 8 in]
        n201 = call <vilib>:"Set Intensity Graph Value.vi"("Value"=w465, "graph_utilities in"=w475) -> ("error out"=w470:errorcluster, "graph_utilities out"=w479:refnum<class "graph_utilities.lvclass">)  [unwired: 8 in]
        n202 = call <vilib>:"Set Intensity Graph Value.vi"("Value"=w465, "graph_utilities in"=w473) -> ("error out"=w468:errorcluster, "graph_utilities out"=w477:refnum<class "graph_utilities.lvclass">)  [unwired: 8 in]
        n203 = call <vilib>:"Set Intensity Graph Value.vi"("Value"=w465, "graph_utilities in"=w472) -> ("error out"=w467:errorcluster, "graph_utilities out"=w476:refnum<class "graph_utilities.lvclass">)  [unwired: 8 in]
        n204 = call-poly <vilib>:"Set XY Graph Value.vi"("error in (no error)"=w463, "XY-data"=w462, "graph_utilities in"=w464) -> ()  [unwired: 7 in, 2 out]
        n205 = call-poly <vilib>:"Set XY Graph Value.vi"("error in (no error)"=w471, "XY-data"=w462, "graph_utilities in"=w480) -> ()  [unwired: 7 in, 2 out]
        n206 = call-poly <vilib>:"Set XY Graph Value.vi"("error in (no error)"=w469, "XY-data"=w462, "graph_utilities in"=w478) -> ()  [unwired: 7 in, 2 out]
        n207 = call-poly <vilib>:"Set XY Graph Value.vi"("error in (no error)"=w470, "XY-data"=w462, "graph_utilities in"=w479) -> ()  [unwired: 7 in, 2 out]
        n208 = call-poly <vilib>:"Set XY Graph Value.vi"("error in (no error)"=w468, "XY-data"=w462, "graph_utilities in"=w477) -> ()  [unwired: 7 in, 2 out]
        n209 = call-poly <vilib>:"Set XY Graph Value.vi"("error in (no error)"=w467, "XY-data"=w462, "graph_utilities in"=w476) -> ()  [unwired: 7 in, 2 out]
        n210 = local write "XY Graph: Antisymmetric"(w462) -> ()
        n211 = local write "XY Graph: Symmetric"(w462) -> ()
        n212 = call <vilib>:"Add State(s) to Queue__jki_lib_state_machine.vi"("State(s) in (\"\")"=w485) -> ("States Out"=w484:string)  [unwired: 14 in]
      }
      frame "Graph: Linecut" {
        # "Do not put any code in this frame.\n(It is a separator no-op. You can make a copy of this frame to create a new Macro frame)"
        n213 = Unbundle By Name(w499) -> ("Graph.Data: Intensity/Vertical"=w498:refnum<class "graph_utilities.lvclass">, "Graph.Data: Intensity/Horizontal"=w497:refnum<class "graph_utilities.lvclass">, "Graph.Differential: Intensity/Vertical"=w496:refnum<class "graph_utilities.lvclass">, "Graph.Differential: Intensity/Horizontal"=w495:refnum<class "graph_utilities.lvclass">)
        n214 = call <vilib>:"Intensity Graph Linecut (Vertical).vi"("error in (no error)"=w492, "width (vertical)"="width (vertical)", "graph_utilities in"=w498) -> ("error out"=w493:errorcluster)  [unwired: 7 in, 1 out]
        n215 = call <vilib>:"Intensity Graph Linecut (Horizontal).vi"("error in (no error)"=w493, "width (horizontal)"="width (horizontal)", "graph_utilities in"=w497) -> ("error out"=w494:errorcluster)  [unwired: 7 in, 1 out]
        n216 = call <vilib>:"Intensity Graph Linecut (Vertical).vi"("error in (no error)"=w494, "width (vertical)"="width (vertical) 2", "graph_utilities in"=w496) -> ("error out"=w491:errorcluster)  [unwired: 7 in, 1 out]
        n217 = call <vilib>:"Intensity Graph Linecut (Horizontal).vi"("error in (no error)"=w491, "width (horizontal)"="width (horizontal) 2", "graph_utilities in"=w495) -> ("error out"=w490:errorcluster)  [unwired: 7 in, 1 out]
        n218 = call <vilib>:"Add State(s) to Queue__jki_lib_state_machine.vi"("State(s) in (\"\")"=w501) -> ("States Out"=w500:string)  [unwired: 14 in]
      }
      frame "Graph: Update Color 1" {
        # "Do not put any code in this frame.\n(It is a separator no-op. You can make a copy of this frame to create a new Macro frame)"
        n219 = Unbundle By Name(w507) -> ("Graph.Data: Intensity/Vertical"=w506:refnum<class "graph_utilities.lvclass">)
        n220 = call <vilib>:"Choose Color Table.vi"("Color Map"="Color Map") -> ("Color Table"=w505:u32[])  [unwired: 7 in, 3 out]
        n221 = call <vilib>:"Set Intensity Graph Z Color.vi"("error in (no error)"=w502, "Colors []"=w505, "graph_utilities in"=w506) -> ("error out"=w503:errorcluster)  [unwired: 7 in, 1 out]
        n222 = call <vilib>:"Add State(s) to Queue__jki_lib_state_machine.vi"("State(s) in (\"\")"=w509) -> ("States Out"=w508:string)  [unwired: 14 in]
      }
      frame "Graph: Update Color 2" {
        # "Do not put any code in this frame.\n(It is a separator no-op. You can make a copy of this frame to create a new Macro frame)"
        n223 = Unbundle By Name(w515) -> ("Graph.Differential: Intensity/Vertical"=w513:refnum<class "graph_utilities.lvclass">)
        n224 = call <vilib>:"Choose Color Table.vi"("Color Map"="Color Map 2") -> ("Color Table"=w514:u32[])  [unwired: 7 in, 3 out]
        n225 = call <vilib>:"Set Intensity Graph Z Color.vi"("error in (no error)"=w511, "Colors []"=w514, "graph_utilities in"=w513) -> ("error out"=w512:errorcluster)  [unwired: 7 in, 1 out]
        n226 = call <vilib>:"Add State(s) to Queue__jki_lib_state_machine.vi"("State(s) in (\"\")"=w517) -> ("States Out"=w516:string)  [unwired: 14 in]
      }
      frame "---------- File ----------" {
        # "Do not put any code in this frame.\n(It is a separator no-op. You can make a copy of this frame to create a new Macro frame)"
        n227 = call <vilib>:"Add State(s) to Queue__jki_lib_state_machine.vi"("State(s) in (\"\")"=w521) -> ("States Out"=w520:string)  [unwired: 14 in]
      }
      frame "File: Load Metadata" {
        # "Do not put any code in this frame.\n(It is a separator no-op. You can make a copy of this frame to create a new Macro frame)"
        n228 = Unbundle By Name(w536) -> ("Rings"=w529:T10, "Path"=w524:path)
        n229 = Empty String/Path?(string/path=w524) -> (empty?=w523:bool)
        n230 = case shown="\"TDMS\"" "Data Type" {
          tunnel: ["*.itx" ("pattern") "*.dat" ("pattern") "*.tdms" ("pattern")] -> w525
          frame Default {
          }
          frame "DAT" {
          }
          frame "TDMS" {
          }
        }
        n231 = case shown="False" w523 {
          tunnel: [w549 _] -> w534
          tunnel: [w548 w558] -> w533
          tunnel: [w547 "" ("Notes")] -> w527
          tunnel: w526 -> [w545 w558]
          tunnel: w525 -> [w543 _]
          tunnel: w524 -> [w542 _]
          frame False {
            n232 = File/Directory Info(path=w542, error in=w545) -> (path out=w540:path, directory=w541:bool, error out=w539:errorcluster)  [unwired: 4 out]
            n233 = case shown="True" w541 {
              tunnel: w540 -> [w551 w556]
              tunnel: [w551 w552] -> w546
              tunnel: w539 -> [w550 w555]
              tunnel: [w550 w554] -> w544
              tunnel: w543 -> [_ w553]
              frame False {
              }
              frame True {
                n234 = call <vilib>:"Recursive File List.vi"("pattern"=w553, "error in (no error)"=w555, "Folder Path"=w556) -> ("error out"=w554:errorcluster, "All Files in Dir"=w557:path[])  [unwired: 4 in, 3 out]
                n235 = Index Array(array=w557) -> (element=w552:path)  [unwired: 1 in]
              }
            }
            n236 = call <userlib>:"Data Read.vi"("error in (no error)"=w544, "path"=w546) -> ("error out"=w548:errorcluster, "Notes"=w547:string, "Data (Dictionary)"=w549:T6[])  [unwired: 6 in, 1 out]
          }
          frame True {
          }
        }
        "Notes" <- w527
        n237 = Cluster To Array(cluster=w529) -> (array=w528:refnum<vi>[])
        n238 = call "List Map Keys and Values.vim"("error in (no error)"=w533, "map in"=w534) -> ("error out"=w532:errorcluster, "Keys"=w535:string[])  [unwired: 6 in, 2 out]
        n239 = for {
          tunnel: w535 -> [w566]
          tunnel: w532 -> [w565]
          tunnel: [w564] -> w531 mode=indexing
          tunnel: w528 -> [w563] mode=indexing
          # "populate ring with channel names"
          n240 = call <userlib>:"Populate Ring Text [].vi"("error in (no error)"=w565, "Strings []"=w566, "Ring in"=w563) -> ("error out"=w564:errorcluster)  [unwired: 8 in]
        }
        n241 = Merge Errors(w531) -> (w530:errorcluster)
        n242 = call <vilib>:"Add State(s) to Queue__jki_lib_state_machine.vi"("State(s) in (\"\")"=w538) -> ("States Out"=w537:string)  [unwired: 14 in]
      }
      frame "File: List Folder" {
        # "File: Load\n(Add code here for loading your data)"
        n243 = local read "Data Type"() -> (w567:T1)
        n244 = Unbundle By Name(w576) -> ("Path"=w575:path)
        n245 = File/Directory Info(path=w575, error in=w574) -> (path out=w570:path, directory=w569:bool, error out=w571:errorcluster)  [unwired: 4 out]
        n246 = case shown="\"TDMS\"" w567 {
          tunnel: ["*.itx" ("pattern") "*.dat" ("pattern") "*.tdms" ("pattern")] -> w573
          frame Default {
          }
          frame "DAT" {
          }
          frame "TDMS" {
          }
        }
        n247 = case shown="True" w569 {
          tunnel: w570 -> [w582 w588]
          tunnel: [w580 w584] -> w572
          tunnel: w571 -> [w581 w587]
          tunnel: [w581 w586] -> w568
          tunnel: w573 -> [_ w585]
          frame False {
            n248 = Build Array(w582) -> (w580:path[])
          }
          frame True {
            n249 = case shown="False" "list recursive" {
              tunnel: w588 -> [w595 w600]
              tunnel: w587 -> [w594 w599]
              tunnel: [w590 w598] -> w586
              tunnel: w585 -> [w589 w597]
              tunnel: [w591 w596] -> w584
              frame False {
                n250 = List Folder(path=w595, pattern=w589, error in=w594) -> (path out=w593:path, filenames=w592:string[], error out=w590:errorcluster)  [unwired: 1 in, 1 out]
                n251 = call-poly <userlib>:"Build Path__ogtk.vi"("name or relative path"=w592, "base path"=w593) -> ("appended path"=w591:path[])
              }
              frame True {
                n252 = call <vilib>:"Recursive File List.vi"("pattern"=w597, "error in (no error)"=w599, "Folder Path"=w600) -> ("error out"=w598:errorcluster, "All Files in Dir"=w596:path[])  [unwired: 4 in, 3 out]
              }
            }
          }
        }
        n253 = Bundle By Name(cluster=w576, "Paths"=w572) -> (w577:T7)
        n254 = call <vilib>:"Add State(s) to Queue__jki_lib_state_machine.vi"("State(s) in (\"\")"=w579) -> ("States Out"=w578:string)  [unwired: 14 in]
      }
      frame "File: Load" {
        # "File: Load\n(Add code here for loading your data)"
        n255 = Unbundle By Name(w611) -> ("Paths"=w607:path[])
        n256 = Empty Array?(array=w607) -> (empty?=w610:bool)
        n257 = case shown="False" w610 {
          tunnel: [_ cluster{"Intensity Data":dbl[], "Array":dbl[]}[] [{"Intensity Data"=[0.0, 0.004, 0.008, 0.012, 0.016, 0.02, 0.024, 0.028, 0.032, 0.036000000000000004, 0.04, 0.044, 0.048, 0.052000000000000005, 0.056, 0.06, 0.064, 0.068, 0.07200000000000001, 0.076, 0.08, 0.084, 0.088, 0.092, 0.096, 0.1, 0.10400000000000001, 0.108, 0.112, 0.116, 0.12, 0.124, 0.128, 0.132, 0.136, 0.14, 0.14400000000000002, 0.148, 0.152, 0.156, 0.16, 0.164, 0.168, 0.17200000000000001, 0.176, 0.18, 0.184, 0.188, 0.192, 0.196, 0.2, 0.20400000000000001, 0.20800000000000002, 0.212, 0.216, 0.22, 0.224, 0.228, 0.232, 0.23600000000000002, 0.24, 0.244, 0.248, 0.252, 0.256, 0.26, 0.264, 0.268, 0.272, 0.276, 0.28, 0.28400000000000003, 0.28800000000000003, 0.292, 0.296, 0.3, 0.304, 0.308, 0.312, 0.316, 0.32, 0.324, 0.328, 0.332, 0.336, 0.34, 0.34400000000000003, 0.34800000000000003, 0.352, 0.356, 0.36, 0.364, 0.368, 0.372, 0.376, 0.38, 0.384, 0.388, 0.392, 0.396, 0.4, 0.404, 0.40800000000000003, 0.41200000000000003, 0.41600000000000004, 0.42, 0.424, 0.428, 0.432, 0.436, 0.44, 0.444, 0.448, 0.452, 0.456, 0.46, 0.464, 0.468, 0.47200000000000003, 0.47600000000000003, 0.48, 0.484, 0.488, 0.492, 0.496, 0.5, 0.504, 0.508, 0.512, 0.516, 0.52, 0.524, 0.528, 0.532, 0.536, 0.54, 0.544, 0.548, 0.552, 0.556, 0.56, 0.5640000000000001, 0.5680000000000001, 0.5720000000000001, 0.5760000000000001, 0.58, 0.584, 0.588, 0.592, 0.596, 0.6, 0.604, 0.608, 0.612, 0.616, 0.62, 0.624, 0.628, 0.632, 0.636, 0.64, 0.644, 0.648, 0.652, 0.656, 0.66, 0.664, 0.668, 0.672, 0.676, 0.68, 0.684, 0.6880000000000001, 0.6920000000000001, 0.6960000000000001, 0.7000000000000001, 0.704, 0.708, 0.712, 0.716, 0.72, 0.724, 0.728, 0.732, 0.736, 0.74, 0.744, 0.748, 0.752, 0.756, 0.76, 0.764, 0.768, 0.772, 0.776, 0.78, 0.784, 0.788, 0.792, 0.796, 0.8, 0.804, 0.808, 0.812, 0.8160000000000001, 0.8200000000000001, 0.8240000000000001, 0.8280000000000001, 0.8320000000000001, 0.836, 0.84, 0.844, 0.848, 0.852, 0.856, 0.86, 0.864, 0.868, 0.872, 0.876, 0.88], "Array"=[1.68063e-07, 1.37198e-07, 8.79687e-08, 1.06463e-07, 1.07999e-07, 1.50443e-07, 1.6136e-07, 1.60216e-07, 1.51628e-07, 1.62347e-07, 2.24052e-07, 2.12498e-07, 1.69888e-07, 2.07771e-07, 2.10504e-07, 1.16164e-07, 1.03648e-07, 1.88353e-07, 2.52956e-07, 1.81322e-07, 1.3598e-07, 1.93502e-07, 3.06623e-07, 1.81397e-07, 1.56136e-07, 7.65771e-08, 1.0323e-07, 2.25052e-07, 2.18994e-07, 1.48687e-07, 1.23465e-07, 1.94812e-07, 8.89733e-08, 1.01215e-07, 1.91375e-07, 1.83998e-07, 1.70281e-07, 2.66741e-07, 1.84557e-07, 1.35922e-07, 1.53284e-07, 1.28241e-07, 1.84801e-07, 1.04068e-07, 8.03285e-08, 1.04402e-07, 8.12206e-08, 5.15301e-08, 2.02427e-07, 1.78907e-07, 1.0348e-07, 8.96397e-08, 1.49064e-07, 2.10614e-07, 1.94321e-07, 1.23458e-07, 2.49381e-08, 1.85551e-07, 1.98644e-07, 2.30779e-07, 3.77495e-07, 6.72036e-07, 1.17947e-06, 1.75588e-06, 2.53801e-06, 3.50995e-06, 4.10398e-06, 4.4421e-06, 4.54957e-06, 4.46684e-06, 4.29614e-06, 4.03689e-06, 3.7785e-06, 3.52652e-06, 3.3015e-06, 3.0176e-06, 2.73351e-06, 2.48081e-06, 2.28944e-06, 2.06704e-06, 1.80961e-06, 1.62787e-06, 1.44499e-06, 1.27341e-06, 1.12003e-06, 1.00442e-06, 8.63595e-07, 7.29893e-07, 6.0347e-07, 5.41881e-07, 4.90755e-07, 4.14075e-07, 3.64346e-07, 3.41478e-07, 3.11551e-07, 2.93279e-07, 3.09014e-07, 3.23829e-07, 3.14767e-07, 3.13298e-07, 3.2943e-07, 3.73559e-07, 3.85052e-07, 4.12776e-07, 4.52513e-07, 4.63779e-07, 5.00565e-07, 5.25226e-07, 5.28226e-07, 5.09122e-07, 4.69838e-07, 4.77525e-07, 4.87608e-07, 4.64681e-07, 4.29366e-07, 4.10075e-07, 3.911e-07, 3.53091e-07, 3.11529e-07, 2.80052e-07, 2.48962e-07, 2.2069e-07, 2.00389e-07, 1.80056e-07, 1.71025e-07, 1.52747e-07, 1.20455e-07, 1.10317e-07, 1.22804e-07, 1.19285e-07, 1.05556e-07, 1.00514e-07, 1.16004e-07, 1.33715e-07, 1.48638e-07, 1.67858e-07, 1.60768e-07, 1.72191e-07, 1.90163e-07, 2.12957e-07, 2.27031e-07, 2.42395e-07, 2.5957e-07, 2.75457e-07, 2.81378e-07, 2.87991e-07, 2.8598e-07, 2.99029e-07, 3.10983e-07, 2.98582e-07, 2.92597e-07, 2.96466e-07, 2.75316e-07, 2.60924e-07, 2.73094e-07, 2.76228e-07, 2.69051e-07, 2.49348e-07, 2.40239e-07, 2.38694e-07, 2.46997e-07, 2.3754e-07, 2.31936e-07, 2.37921e-07, 2.4129e-07, 2.36577e-07, 2.27175e-07, 2.23179e-07, 2.32753e-07, 2.22017e-07, 2.21659e-07, 2.35338e-07, 2.45551e-07, 2.48375e-07, 2.61624e-07, 2.68417e-07, 2.63606e-07, 2.83272e-07, 2.96328e-07, 2.89196e-07, 2.96568e-07, 3.03707e-07, 3.06523e-07, 3.1915e-07, 3.12655e-07, 2.95357e-07, 2.95008e-07, 2.98448e-07, 3.09012e-07, 3.01923e-07, 2.96206e-07, 3.10244e-07, 3.04155e-07, 2.92192e-07, 2.85057e-07, 2.82269e-07, 2.90168e-07, 2.75276e-07, 2.42554e-07, 2.36848e-07, 2.39448e-07, 2.14838e-07, 2.06682e-07, 2.0462e-07, 1.85893e-07, 1.77192e-07, 1.71389e-07, 1.56772e-07, 1.51419e-07, 1.47796e-07, 1.53989e-07, 1.38128e-07, 1.40478e-07, 1.52301e-07, 1.42379e-07, 1.31716e-07, 1.3604e-07, 1.51662e-07, 1.43388e-07, 1.35586e-07, 1.45146e-07]}, ...(73 in all)] ("Vertical")] -> w604
          tunnel: [w615 dbl[] [-9.0, -8.75, -8.5, -8.25, -8.0, -7.75, -7.5, -7.25, -7.0, -6.75, -6.5, -6.25, -6.0, -5.75, -5.5, -5.25, -5.0, -4.75, -4.5, -4.25, -4.0, -3.75, -3.5, -3.25, -3.0, -2.75, -2.5, -2.25, -2.0, -1.75, -1.5, -1.25, -1.0, -0.75, -0.5, -0.25, 0.0, 0.25, 0.5, 0.75, 1.0, 1.25, 1.5, 1.75, 2.0, 2.25, 2.5, 2.75, 3.0, 3.25, 3.5, 3.75, 4.0, 4.25, 4.5, 4.75, 5.0, 5.25, 5.5, 5.75, 6.0, 6.25, 6.5, 6.75, 7.0, 7.25, 7.5, 7.75, 8.0, 8.25, 8.5, 8.75, 9.0] ("X")] -> w608
          tunnel: [w620 _] -> w609
          tunnel: w607 -> [w618 _]
          tunnel: w606 -> [w617 w641]
          tunnel: [w619 w641] -> w605
          frame False {
            n258 = for {
              tunnel: [w633] -> w621 mode=indexing
              tunnel: w617 -> [w631]
              tunnel: [w630] -> w616
              tunnel: w618 -> [w625] mode=indexing
              tunnel: [w623] -> w615 mode=indexing
              n259 = Strip Path(path=w625) -> (name=w629:string)  [unwired: 1 out]
              n260 = call <userlib>:"Data Read.vi"("Append Index"=-1, "error in (no error)"=w631, "path"=w625) -> ("error out"=w630:errorcluster, "Notes"=w624:string, "Data (Dictionary)"=w632:T6[])  [unwired: 5 in, 1 out]
              n261 = Format Into String(format string="Loading %s", w629) -> (resulting string=w627:string)  [unwired: 2 in, 1 out]
              n262 = local write "Current State"(w627) -> ()
              n263 = Bundle("Data (Dictionary)"=w632) -> (w633:cluster{"Data (Dictionary)":T6[]})  [unwired: 1 in]
              n264 = case shown="True" "param in notes" {
                tunnel: w624 -> [_ w640]
                tunnel: [0.0 w639] -> w623
                frame False {
                }
                frame True {
                  n265 = Match Pattern(string=w640, regular expression="regex before") -> (after substring=w637:string)  [unwired: 1 in, 3 out]
                  n266 = Match Pattern(string=w637, regular expression="regex after") -> (before substring=w636:string)  [unwired: 1 in, 3 out]
                  n267 = Fract/Exp String To Number(string=w636) -> (number=w639:dbl)  [unwired: 3 in, 1 out]
                }
              }
            }
            n268 = call <userlib>:"Variant to Dictionary.vi"("error in (no error)"=w616, "Array in"=w621) -> ("error out"=w619:errorcluster, "Array out"=w620:cluster{"Data (Dictionary)":T6[]}[])  [unwired: 8 in]
          }
          frame True {
            # "Demonstration Data"
          }
        }
        n269 = Bundle By Name(cluster=w611, "XY Data (unprocessed)"=w604, "XY Data (processed 1)"=w604, "XY Data (processed 2)"=w604, "Parameter"=w608, "Dictionaries"=w609) -> (w612:T7)
        n270 = call <vilib>:"Add State(s) to Queue__jki_lib_state_machine.vi"("State(s) in (\"\")"=w614) -> ("States Out"=w613:string)  [unwired: 14 in]
      }
      frame "File: Save" {
        # "Do not put any code in this frame.\n(It is a separator no-op. You can make a copy of this frame to create a new Macro frame)"
        n271 = Unbundle By Name(w650) -> ("Path"=w649:path)
        n272 = Strip Path(path=w649) -> (stripped path=w646:path)  [unwired: 1 out]
        n273 = control-ref of="XY Graph: Processed"() -> (w651:refnum<vi>)
        n274 = Build Path(base path=w646, name or relative path="export\\export.tx") -> (appended path=w644:path)
        n275 = call <userlib>:"XY Graph to Igor Graph.vi"("error in (no error)"=w647, "XY Graph Reference"=w651, "Path"=w644) -> ("error out"=w648:errorcluster)  [unwired: 7 in, 1 out]
        n276 = call <vilib>:"Add State(s) to Queue__jki_lib_state_machine.vi"("State(s) in (\"\")"=w653) -> ("States Out"=w652:string)  [unwired: 14 in]
      }
      frame "---------- XY ----------" {
        # "Template Separator\n(You can make a copy of, or modify, this frame)"
        n277 = Unbundle By Name(w658) -> ("XY Data (processed 1)"=w659:cluster{"X-array":dbl[], "Y-array":dbl[]}[])
        n278 = call-poly <vilib>:"Add.vi"("error in (no error)"=w655, "XY-data"=w659) -> ("error out"=w654:errorcluster, "XY-data out"=w656:cluster{"X-array":dbl[], "Y-array":dbl[]}[])  [unwired: 8 in]
        n279 = Bundle By Name(cluster=w658, "XY Data (processed 1)"=w656) -> (w657:T7)
        n280 = call <vilib>:"Add State(s) to Queue__jki_lib_state_machine.vi"("State(s) in (\"\")"=w661) -> ("States Out"=w660:string)  [unwired: 14 in]
      }
      frame "XY: Add" {
        # "XY: Add\n(You can make a copy of, or modify, this frame)"
        n281 = Unbundle By Name(w668) -> ("XY Data (processed 1)"=w669:cluster{"X-array":dbl[], "Y-array":dbl[]}[])
        n282 = call-poly <vilib>:"Add.vi"("error in (no error)"=w665, "y (0)"="y", "x (0)"="x", "XY-data"=w669) -> ("error out"=w664:errorcluster, "XY-data out"=w666:cluster{"X-array":dbl[], "Y-array":dbl[]}[])  [unwired: 6 in]
        n283 = Bundle By Name(cluster=w668, "XY Data (processed 1)"=w666) -> (w667:T7)
        n284 = call <vilib>:"Add State(s) to Queue__jki_lib_state_machine.vi"("State(s) in (\"\")"=w671) -> ("States Out"=w670:string)  [unwired: 14 in]
      }
      frame "XY: Subtract" {
        # "Template Separator\n(You can make a copy of, or modify, this frame)"
        n285 = Unbundle By Name(w678) -> ("XY Data (processed 1)"=w679:cluster{"X-array":dbl[], "Y-array":dbl[]}[])
        n286 = local read "x"() -> (w672:dbl)
        n287 = local read "y"() -> (w673:dbl)
        n288 = call-poly <vilib>:"Subtract.vi"("error in (no error)"=w675, "y (0)"=w673, "x (0)"=w672, "XY-data"=w679) -> ("error out"=w674:errorcluster, "XY-data out"=w676:cluster{"X-array":dbl[], "Y-array":dbl[]}[])  [unwired: 6 in]
        n289 = Bundle By Name(cluster=w678, "XY Data (processed 1)"=w676) -> (w677:T7)
        n290 = call <vilib>:"Add State(s) to Queue__jki_lib_state_machine.vi"("State(s) in (\"\")"=w681) -> ("States Out"=w680:string)  [unwired: 14 in]
      }
      frame "XY: Multiply" {
        # "Template Separator\n(You can make a copy of, or modify, this frame)"
        n291 = Unbundle By Name(w688) -> ("XY Data (processed 1)"=w689:cluster{"X-array":dbl[], "Y-array":dbl[]}[])
        n292 = local read "x"() -> (w683:dbl)
        n293 = local read "y"() -> (w682:dbl)
        n294 = call-poly <vilib>:"Multiply.vi"("error in (no error)"=w685, "y (1)"=w682, "x (1)"=w683, "XY-data"=w689) -> ("error out"=w684:errorcluster, "XY-data out"=w686:cluster{"X-array":dbl[], "Y-array":dbl[]}[])  [unwired: 6 in]
        n295 = Bundle By Name(cluster=w688, "XY Data (processed 1)"=w686) -> (w687:T7)
        n296 = call <vilib>:"Add State(s) to Queue__jki_lib_state_machine.vi"("State(s) in (\"\")"=w691) -> ("States Out"=w690:string)  [unwired: 14 in]
      }
      frame "XY: Square" {
        # "Template Separator\n(You can make a copy of, or modify, this frame)"
        n297 = Unbundle By Name(w696) -> ("XY Data (processed 1)"=w697:cluster{"X-array":dbl[], "Y-array":dbl[]}[])
        n298 = call-poly <vilib>:"Square.vi"("error in (no error)"=w693, "XY-data"=w697) -> ("error out"=w692:errorcluster, "XY-data out"=w694:cluster{"X-array":dbl[], "Y-array":dbl[]}[])  [unwired: 8 in]
        n299 = Bundle By Name(cluster=w696, "XY Data (processed 1)"=w694) -> (w695:T7)
        n300 = call <vilib>:"Add State(s) to Queue__jki_lib_state_machine.vi"("State(s) in (\"\")"=w699) -> ("States Out"=w698:string)  [unwired: 14 in]
      }
      frame "XY: Log" {
        # "Template Separator\n(You can make a copy of, or modify, this frame)"
        n301 = Unbundle By Name(w704) -> ("XY Data (processed 1)"=w701:cluster{"X-array":dbl[], "Y-array":dbl[]}[])
        n302 = for {
          tunnel: w701 -> [w710] mode=indexing
          tunnel: [w709] -> w700 mode=indexing
          n303 = Unbundle By Name(w710) -> ("Y-array"=w708:dbl[])
          n304 = Natural Logarithm(1:w708) -> (0:w707:dbl[])
          n305 = Bundle By Name(cluster=w710, "Y-array"=w707) -> (w709:cluster{"X-array":dbl[], "Y-array":dbl[]})
        }
        n306 = Bundle By Name(cluster=w704, "XY Data (processed 1)"=w700) -> (w703:T7)
        n307 = call <vilib>:"Add State(s) to Queue__jki_lib_state_machine.vi"("State(s) in (\"\")"=w706) -> ("States Out"=w705:string)  [unwired: 14 in]
      }
      frame "XY: Divide" {
        # "Template Separator\n(You can make a copy of, or modify, this frame)"
        n308 = Unbundle By Name(w717) -> ("XY Data (processed 1)"=w718:cluster{"X-array":dbl[], "Y-array":dbl[]}[])
        n309 = local read "x"() -> (w712:dbl)
        n310 = local read "y"() -> (w711:dbl)
        n311 = call-poly <vilib>:"Divide.vi"("error in (no error)"=w714, "y (1)"=w711, "x (1)"=w712, "XY-data"=w718) -> ("error out"=w713:errorcluster, "XY-data out"=w715:cluster{"X-array":dbl[], "Y-array":dbl[]}[])  [unwired: 6 in]
        n312 = Bundle By Name(cluster=w717, "XY Data (processed 1)"=w715) -> (w716:T7)
        n313 = call <vilib>:"Add State(s) to Queue__jki_lib_state_machine.vi"("State(s) in (\"\")"=w720) -> ("States Out"=w719:string)  [unwired: 14 in]
      }
      frame "XY: Sort" {
        # "Template Separator\n(You can make a copy of, or modify, this frame)"
        n314 = Unbundle By Name(w725) -> ("XY Data (processed 1)"=w726:cluster{"X-array":dbl[], "Y-array":dbl[]}[])
        n315 = call-poly <vilib>:"Sort.vi"("error in (no error)"=w722, "XY-data"=w726) -> ("error out"=w721:errorcluster, "Sorted XY-data out"=w723:cluster{"X-array":dbl[], "Y-array":dbl[]}[])  [unwired: 7 in, 1 out]
        n316 = Bundle By Name(cluster=w725, "XY Data (processed 1)"=w723) -> (w724:T7)
        n317 = call <vilib>:"Add State(s) to Queue__jki_lib_state_machine.vi"("State(s) in (\"\")"=w728) -> ("States Out"=w727:string)  [unwired: 14 in]
      }
      frame "XY: Decimate" {
        # "Template Separator\n(You can make a copy of, or modify, this frame)"
        n318 = Unbundle By Name(w735) -> ("XY Data (processed 1)"=w736:cluster{"X-array":dbl[], "Y-array":dbl[]}[])
        n319 = call-poly <vilib>:"Decimate.vi"("error in (no error)"=w732, "averaging (off)"="averaging", "decimating factor (1)"="decimating factor", "XY-data"=w736) -> ("error out"=w731:errorcluster, "Decimated XY-data out"=w733:cluster{"X-array":dbl[], "Y-array":dbl[]}[])  [unwired: 6 in]
        n320 = Bundle By Name(cluster=w735, "XY Data (processed 1)"=w733) -> (w734:T7)
        n321 = call <vilib>:"Add State(s) to Queue__jki_lib_state_machine.vi"("State(s) in (\"\")"=w738) -> ("States Out"=w737:string)  [unwired: 14 in]
      }
      frame "XY: Swap" {
        # "Template Separator\n(You can make a copy of, or modify, this frame)"
        n322 = Unbundle By Name(w743) -> ("XY Data (processed 1)"=w744:cluster{"X-array":dbl[], "Y-array":dbl[]}[])
        n323 = call-poly <vilib>:"Swap X and Y.vi"("error in (no error)"=w740, "XY-data"=w744) -> ("error out"=w739:errorcluster, "XY-data out"=w741:cluster{"X-array":dbl[], "Y-array":dbl[]}[])  [unwired: 8 in]
        n324 = Bundle By Name(cluster=w743, "XY Data (processed 1)"=w741) -> (w742:T7)
        n325 = call <vilib>:"Add State(s) to Queue__jki_lib_state_machine.vi"("State(s) in (\"\")"=w746) -> ("States Out"=w745:string)  [unwired: 14 in]
      }
      frame "XY: Reverse" {
        # "Template Separator\n(You can make a copy of, or modify, this frame)"
        n326 = Unbundle By Name(w751) -> ("XY Data (processed 1)"=w752:cluster{"X-array":dbl[], "Y-array":dbl[]}[])
        n327 = call-poly <vilib>:"Reverse.vi"("error in (no error)"=w748, "XY-data"=w752) -> ("error out"=w747:errorcluster, "Reversed XY-data out"=w749:cluster{"X-array":dbl[], "Y-array":dbl[]}[])  [unwired: 8 in]
        n328 = Bundle By Name(cluster=w751, "XY Data (processed 1)"=w749) -> (w750:T7)
        n329 = call <vilib>:"Add State(s) to Queue__jki_lib_state_machine.vi"("State(s) in (\"\")"=w754) -> ("States Out"=w753:string)  [unwired: 14 in]
      }
      frame "XY: Subset" {
        # "Template Separator\n(You can make a copy of, or modify, this frame)"
        n330 = case shown="\"\"" w755 {
          selector: w755 -> [w768 _]
          tunnel: [w766 "Method"] -> w757
          frame Default {
            n331 = Scan From String(input string=w768, default 1=enum16{"Slider (%)", "X[] min and max"}."X[] min and max" ("Method")) -> (output 1=w766:enum16{"Slider (%)", "X[] min and max"})  [unwired: 3 in, 3 out]
          }
          frame "" {
          }
        }
        n332 = Unbundle By Name(w762) -> ("XY Data (processed 1)"=w763:cluster{"X-array":dbl[], "Y-array":dbl[]}[])
        n333 = call-poly <vilib>:"Subset.vi"("error in (no error)"=w759, "Subset Method"=w757, "Subset Slider"="Subset Slider", "XY-data"=w763) -> ("error out"=w758:errorcluster, "Subset XY-data out"=w760:cluster{"X-array":dbl[], "Y-array":dbl[]}[])  [unwired: 6 in]
        n334 = Bundle By Name(cluster=w762, "XY Data (processed 1)"=w760) -> (w761:T7)
        n335 = call <vilib>:"Add State(s) to Queue__jki_lib_state_machine.vi"("State(s) in (\"\")"=w765) -> ("States Out"=w764:string)  [unwired: 14 in]
      }
      frame "XY: Derivative" {
        # "Template Separator\n(You can make a copy of, or modify, this frame)"
        n336 = Unbundle By Name(w775) -> ("XY Data (processed 1)"=w776:cluster{"X-array":dbl[], "Y-array":dbl[]}[])
        n337 = call-poly <vilib>:"Derivative.vi"("error in (no error)"=w773, "Type"="Type", "XY-data"=w776) -> ("error out"=w772:errorcluster, "Differential out"=w770:cluster{"X-array":dbl[], "Y-array":dbl[]}[])  [unwired: 6 in, 1 out]
        n338 = Bundle By Name(cluster=w775, "XY Data (processed 1)"=w770) -> (w774:T7)
        n339 = call <vilib>:"Add State(s) to Queue__jki_lib_state_machine.vi"("State(s) in (\"\")"=w778) -> ("States Out"=w777:string)  [unwired: 14 in]
      }
      frame "XY: Difference Quotient" {
        # "Template Separator\n(You can make a copy of, or modify, this frame)"
        n340 = Unbundle By Name(w786) -> ("XY Data (processed 1)"=w787:cluster{"X-array":dbl[], "Y-array":dbl[]}[])
        n341 = call-poly <vilib>:"Difference Quotient.vi"("Interval Units (points)"="Units", "error in (no error)"=w784, "Type"="Type", "Window [h] (2)"="Window", "XY-data"=w787) -> ("error out"=w783:errorcluster, "Difference Quotient"=w782:cluster{"X-array":dbl[], "Y-array":dbl[]}[])  [unwired: 4 in, 1 out]
        n342 = Bundle By Name(cluster=w786, "XY Data (processed 1)"=w782) -> (w785:T7)
        n343 = call <vilib>:"Add State(s) to Queue__jki_lib_state_machine.vi"("State(s) in (\"\")"=w789) -> ("States Out"=w788:string)  [unwired: 14 in]
      }
      frame "XY: Interpolate" {
        # "Template Separator\n(You can make a copy of, or modify, this frame)"
        n344 = Unbundle By Name(w795) -> ("XY Data (processed 1)"=w796:cluster{"X-array":dbl[], "Y-array":dbl[]}[])
        n345 = call-poly <vilib>:"Interpolate.vi"("error in (no error)"=w792, "Configure"="Configure", "XY-data"=w796) -> ("error out"=w791:errorcluster, "Interpolated XY-data out"=w793:cluster{"X-array":dbl[], "Y-array":dbl[]}[])  [unwired: 7 in]
        n346 = Bundle By Name(cluster=w795, "XY Data (processed 1)"=w793) -> (w794:T7)
        n347 = call <vilib>:"Add State(s) to Queue__jki_lib_state_machine.vi"("State(s) in (\"\")"=w798) -> ("States Out"=w797:string)  [unwired: 14 in]
      }
      frame "XY: FFT Spectrum" {
        # "Template Separator\n(You can make a copy of, or modify, this frame)"
        n348 = Unbundle By Name(w803) -> ("XY Data (processed 1)"=w804:cluster{"X-array":dbl[], "Y-array":dbl[]}[])
        n349 = call-poly <vilib>:"FFT Spectrum.vi"("error in (no error)"=w800, "XY-data"=w804) -> ("error out"=w799:errorcluster, "XY-data out"=w801:cluster{"X-array":dbl[], "Y-array":dbl[]}[])  [unwired: 6 in, 2 out]
        n350 = Bundle By Name(cluster=w803, "XY Data (processed 1)"=w801) -> (w802:T7)
        n351 = call <vilib>:"Add State(s) to Queue__jki_lib_state_machine.vi"("State(s) in (\"\")"=w806) -> ("States Out"=w805:string)  [unwired: 14 in]
      }
      frame "XY: FFT Power Spectrum" {
        # "Template Separator\n(You can make a copy of, or modify, this frame)"
        n352 = Unbundle By Name(w811) -> ("XY Data (processed 1)"=w812:cluster{"X-array":dbl[], "Y-array":dbl[]}[])
        n353 = call-poly <vilib>:"FFT Power Spectrum.vi"("error in (no error)"=w809, "XY-data"=w812) -> ("error out"=w808:errorcluster, "XY-data out"=w807:cluster{"X-array":dbl[], "Y-array":dbl[]}[])  [unwired: 7 in, 1 out]
        n354 = Bundle By Name(cluster=w811, "XY Data (processed 1)"=w807) -> (w810:T7)
        n355 = call <vilib>:"Add State(s) to Queue__jki_lib_state_machine.vi"("State(s) in (\"\")"=w814) -> ("States Out"=w813:string)  [unwired: 14 in]
      }
      frame "XY: Resample" {
        # "Template Separator\n(You can make a copy of, or modify, this frame)"
        n356 = Unbundle By Name(w819) -> ("XY Data (processed 1)"=w820:cluster{"X-array":dbl[], "Y-array":dbl[]}[])
        n357 = call-poly <vilib>:"Resample.vi"("error in (no error)"=w816, "XY-data"=w820) -> ("error out"=w815:errorcluster, "Resampled XY-data out"=w817:cluster{"X-array":dbl[], "Y-array":dbl[]}[])  [unwired: 8 in]
        n358 = Bundle By Name(cluster=w819, "XY Data (processed 1)"=w817) -> (w818:T7)
        n359 = call <vilib>:"Add State(s) to Queue__jki_lib_state_machine.vi"("State(s) in (\"\")"=w822) -> ("States Out"=w821:string)  [unwired: 14 in]
      }
      frame "XY: Average" {
        # "Template Separator\n(You can make a copy of, or modify, this frame)"
        n360 = Unbundle By Name(w827) -> ("XY Data (processed 1)"=w828:cluster{"X-array":dbl[], "Y-array":dbl[]}[])
        n361 = call <vilib>:"Average.vi"("error in (no error)"=w824, "XY-data"=w828) -> ("error out"=w823:errorcluster, "XY-data out"=w825:cluster{"X-array":dbl[], "Y-array":dbl[]}[])  [unwired: 7 in, 1 out]
        n362 = Bundle By Name(cluster=w827, "XY Data (processed 1)"=w825) -> (w826:T7)
        n363 = call <vilib>:"Add State(s) to Queue__jki_lib_state_machine.vi"("State(s) in (\"\")"=w830) -> ("States Out"=w829:string)  [unwired: 14 in]
      }
      frame "XY: Moving Average" {
        # "Template Separator\n(You can make a copy of, or modify, this frame)"
        n364 = Unbundle By Name(w836) -> ("XY Data (processed 1)"=w837:cluster{"X-array":dbl[], "Y-array":dbl[]}[])
        n365 = call-poly <vilib>:"Moving Average.vi"("error in (no error)"=w833, "Window"="Moving Window", "XY-data"=w837) -> ("error out"=w832:errorcluster, "XY-data out"=w834:cluster{"X-array":dbl[], "Y-array":dbl[]}[])  [unwired: 7 in]
        n366 = Bundle By Name(cluster=w836, "XY Data (processed 1)"=w834) -> (w835:T7)
        n367 = call <vilib>:"Add State(s) to Queue__jki_lib_state_machine.vi"("State(s) in (\"\")"=w839) -> ("States Out"=w838:string)  [unwired: 14 in]
      }
      frame "XY: SG Filter" {
        # "Template Separator\n(You can make a copy of, or modify, this frame)"
        n368 = Unbundle By Name(w845) -> ("XY Data (processed 1)"=w846:cluster{"X-array":dbl[], "Y-array":dbl[]}[])
        n369 = call-poly <vilib>:"Savitsky Golay Filter.vi"("error in (no error)"=w842, "side points (6)"="SG side points", "XY-data"=w846) -> ("error out"=w841:errorcluster, "XY-data out"=w843:cluster{"X-array":dbl[], "Y-array":dbl[]}[])  [unwired: 7 in]
        n370 = Bundle By Name(cluster=w845, "XY Data (processed 1)"=w843) -> (w844:T7)
        n371 = call <vilib>:"Add State(s) to Queue__jki_lib_state_machine.vi"("State(s) in (\"\")"=w848) -> ("States Out"=w847:string)  [unwired: 14 in]
      }
      frame "XY: Zero Phase Filter" {
        # "Template Separator\n(You can make a copy of, or modify, this frame)"
        n372 = Unbundle By Name(w854) -> ("XY Data (processed 1)"=w855:cluster{"X-array":dbl[], "Y-array":dbl[]}[])
        n373 = call-poly <vilib>:"Zero Phase Lowpass Filter.vi"("error in (no error)"=w851, "cutoff period (data)"="Zero Phase cutoff", "XY-data"=w855) -> ("error out"=w850:errorcluster, "XY-data out"=w852:cluster{"X-array":dbl[], "Y-array":dbl[]}[])  [unwired: 7 in]
        n374 = Bundle By Name(cluster=w854, "XY Data (processed 1)"=w852) -> (w853:T7)
        n375 = call <vilib>:"Add State(s) to Queue__jki_lib_state_machine.vi"("State(s) in (\"\")"=w857) -> ("States Out"=w856:string)  [unwired: 14 in]
      }
      frame "XY: Symmeterize" {
        # "Template Separator\n(You can make a copy of, or modify, this frame)"
        n376 = Unbundle By Name(w864) -> ("XY Data (processed 1)"=w865:cluster{"X-array":dbl[], "Y-array":dbl[]}[])
        n377 = call-poly <vilib>:"Symmetrize.vi"("error in (no error)"=w861, "XY-data"=w865) -> ("error out"=w860:errorcluster, "Antisymmetric"=→"XY Graph: Antisymmetric":cluster{"X-array":dbl[], dbl[]}[], "Symmetric"=→"XY Graph: Symmetric":cluster{"X-array":dbl[], dbl[]}[], "XY-data out"=w862:cluster{"X-array":dbl[], "Y-array":dbl[]}[])  [unwired: 6 in]
        n378 = Bundle By Name(cluster=w864, "XY Data (processed 1)"=w862) -> (w863:T7)
        n379 = call <vilib>:"Add State(s) to Queue__jki_lib_state_machine.vi"("State(s) in (\"\")"=w867) -> ("States Out"=w866:string)  [unwired: 14 in]
      }
    }
  }
  n380 = disable-structure shown="Enabled" {
    frame Disabled {
      # "LV-Data API"
      n381 = call "List Map Keys and Values.vim"() -> ()  [unwired: 8 in, 4 out]
      n382 = call <userlib>:"Data Read.vi"() -> ()  [unwired: 8 in, 4 out]
      n383 = call "List Map Keys and Values.vim"() -> ()  [unwired: 8 in, 4 out]
      n384 = call-poly <userlib>:"XY-Data to Dictionary.vi"() -> ()  [unwired: 10 in, 2 out]
      n385 = call <userlib>:"Variant to DBL Array.vi"() -> ()  [unwired: 9 in, 3 out]
      n386 = call "Convert Dictionary to Map.vim"() -> ()  [unwired: 10 in, 2 out]
      n387 = call <userlib>:"Variant to String.vi"() -> ()  [unwired: 10 in, 2 out]
    }
    frame Disabled {
      # "XY-Utilities API"
      n388 = call <vilib>:"Initialize.vi"() -> ()  [unwired: 10 in, 2 out]
      n389 = call-poly <vilib>:"Sort.vi"() -> ()  [unwired: 9 in, 3 out]
      n390 = call-poly <vilib>:"Swap X and Y.vi"() -> ()  [unwired: 10 in, 2 out]
      n391 = call-poly <vilib>:"Difference Quotient.vi"() -> ()  [unwired: 9 in, 3 out]
      n392 = call-poly <vilib>:"Zero Phase Lowpass Filter.vi"() -> ()  [unwired: 10 in, 2 out]
      n393 = call-poly <vilib>:"Add.vi"() -> ()  [unwired: 10 in, 2 out]
      n394 = call <vilib>:"Interpolate Parameter.vi"() -> ()  [unwired: 9 in, 3 out]
      n395 = call-poly <vilib>:"Reverse.vi"() -> ()  [unwired: 10 in, 2 out]
      n396 = call-poly <vilib>:"Get X and Y.vi"() -> ()  [unwired: 8 in, 4 out]
      n397 = call-poly <vilib>:"Derivative.vi"() -> ()  [unwired: 9 in, 3 out]
      n398 = call-poly <vilib>:"Waveform to XY.vi"() -> ()  [unwired: 10 in, 2 out]
      n399 = call-poly <vilib>:"Subtract.vi"() -> ()  [unwired: 10 in, 2 out]
      n400 = call-poly <vilib>:"Moving Average.vi"() -> ()  [unwired: 10 in, 2 out]
      n401 = call-poly <vilib>:"Interpolate.vi"() -> ()  [unwired: 10 in, 2 out]
      n402 = call-poly <vilib>:"Decimate.vi"() -> ()  [unwired: 10 in, 2 out]
      n403 = call-poly <vilib>:"Append.vi"() -> ()  [unwired: 10 in, 2 out]
      n404 = call-poly <vilib>:"XY to Waveform.vi"() -> ()  [unwired: 9 in, 3 out]
      n405 = call-poly <vilib>:"Linear Fit.vi"() -> ()  [unwired: 5 in, 7 out]
      n406 = call-poly <vilib>:"Multiply.vi"() -> ()  [unwired: 10 in, 2 out]
      n407 = call-poly <vilib>:"Savitsky Golay Filter.vi"() -> ()  [unwired: 10 in, 2 out]
      n408 = call-poly <vilib>:"Resample.vi"() -> ()  [unwired: 10 in, 2 out]
      n409 = call <vilib>:"Decimate Array.vi"() -> ()  [unwired: 10 in, 2 out]
      n410 = call-poly <vilib>:"Interpolate Y.vi"() -> ()  [unwired: 9 in, 3 out]
      n411 = call-poly <vilib>:"Divide.vi"() -> ()  [unwired: 10 in, 2 out]
      n412 = call <vilib>:"2D to XY.vi"() -> ()  [unwired: 10 in, 2 out]
      n413 = call-poly <vilib>:"Shift Zero.vi"() -> ()  [unwired: 10 in, 2 out]
      n414 = call-poly <vilib>:"FFT Spectrum.vi"() -> ()  [unwired: 8 in, 4 out]
      n415 = call-poly <vilib>:"Subset.vi"() -> ()  [unwired: 10 in, 2 out]
      n416 = call-poly <vilib>:"Peak Detector.vi"() -> ()  [unwired: 8 in, 4 out]
      n417 = call-poly <vilib>:"Square.vi"() -> ()  [unwired: 10 in, 2 out]
      n418 = call <vilib>:"XY to 2D.vi"() -> ()  [unwired: 8 in, 4 out]
      n419 = call-poly <vilib>:"Remove Outliers.vi"() -> ()  [unwired: 10 in, 2 out]
      n420 = call-poly <vilib>:"Symmetrize.vi"() -> ()  [unwired: 8 in, 4 out]
      n421 = call <vilib>:"Average.vi"() -> ()  [unwired: 9 in, 3 out]
      n422 = call-poly <vilib>:"FFT Power Spectrum.vi"() -> ()  [unwired: 9 in, 3 out]
      n423 = call <vilib>:"Flatten.vi"() -> ()  [unwired: 10 in, 2 out]
      n424 = call-poly <vilib>:"Restrict X Range.vi"() -> ()  [unwired: 10 in, 2 out]
      n425 = call-poly <vilib>:"Log.vi"() -> ()  [unwired: 10 in, 2 out]
    }
    frame Disabled {
      # "Graph Utilities API"
      n426 = call <vilib>:"Intensity Graph to XY Graph (Horizontal).vi"() -> ()  [unwired: 10 in, 2 out]
      n427 = call <vilib>:"XY Graph to Intensity Graph.vi"() -> ()  [unwired: 10 in, 2 out]
      n428 = call <vilib>:"Intensity Graph Linecut (Horizontal).vi"() -> ()  [unwired: 10 in, 2 out]
      n429 = call <vilib>:"Intensity Graph to XY Graph (Vertical).vi"() -> ()  [unwired: 10 in, 2 out]
      n430 = call <vilib>:"Intensity Graph Linecut (Vertical).vi"() -> ()  [unwired: 10 in, 2 out]
    }
    frame Enabled {
    }
  }
